vi "GTcode_v6(reorganized).vi"() -> ()   [LabVIEW 2016]
uses:
  DCScode_simulISS_MAP/flex05-4chPascal.dll
  <vilib>/Utility/config.llb/NI_LVConfig.lvlib
  <vilib>/Utility/config.llb/Write Key (U32).vi
  <vilib>/Utility/config.llb/Read Key (U32).vi
  DCScode_simulISS_MAP/flex05oem8chauto100nsPASCAL_win7.dll
  <vilib>/Analysis/NI_AALBase.lvlib
  <vilib>/Utility/config.llb/Write Key (I32).vi
  <vilib>/Utility/config.llb/Write Key (Double).vi
  <vilib>/Utility/config.llb/Write Key (String).vi
  <vilib>/Utility/config.llb/Read Key (I32).vi
panel:
  in  "Tab\nControl":T1(tab)=enum."Real Time Fitting Parameters" caption="Tab Control"
  out "filtered signal (single sample)":waveform(dbl)(graph)
  out "mean":dbl format="%0.1e"
  out "COV":dbl format="%0.1f"
  in  "Fixed Time":bool
  in  "Detector Used":T2(ring)=enum."Det 2"
  in  "Real Time Fitting?":bool=TRUE
  out "g2":cluster{"Delay Time":sgl[], sgl[]}[](graph) caption="Normalized Correlation Function"
  out "Tau":cluster{"tmp":dbl, dbl}(graph) caption="Relative Changes of Flow"
  in  "QUIT":bool
  in  "Clear plots":bool
  in  "Baseline":bool
  in  "MARK\nMark":bool
  in  "Stop":bool
  in  "Sequence Scan":bool
  out "Mark #":u32
  out "Trial #":u32
  out "Frame #":u32
  out "Det 8":sgl format="%.3f"
  out "Det 7":sgl format="%.3f"
  out "Det 6":sgl format="%.3f"
  out "Det 5":sgl format="%.3f"
  out "Det 4":sgl format="%.3f"
  out "Det 3":sgl format="%.3f"
  out "Det 2":sgl format="%.3f"
  out "Det 1":sgl format="%.3f"
  out "Computer Time":string="2010-1-12 23:16:10"
  in  "D1":bool
  in  "D2":bool
  in  "D3":bool
  in  "D4":bool
  in  "D5":bool
  in  "D6":bool
  in  "D7":bool
  in  "D8":bool
  out "Tau 2":T3(graph)={1.6593152555505744e-08, 3.9427894777554196e-08, 4.065716407938411e-08, 1.5135790977358522e-08, 2.4870420100428357e-08, 7.094765128107397e-08, 0.0, 4.1348620928852906e-07, 1.5886917674344795e-08, 4.0280526032721455e-08, -1.0, -1.0} caption="Blood Flow Index (cm2/s)"
  in  "Fixed # of Frames":u32=5
  out "Status":string="Quit"
  in  "Optical Switch OPEN":bool
  in  "Delay between frames(ms)":u32=500
  out "Time Left (ms)":sgl format="%.3f"
  in  "Integration Time (ms)":sgl=1000.0 min=1 max=13000 step=1
  in  "File Name:":string="test0"
  in  "Data Save Directory:":path=path "C:/data"
  in  "ISS Lasers ON":bool
  in  "Test":bool
  out "Data Levels":dbl(slide) scale=0.0..0.07
  in  "Lines":tag="Dev1/port1/line0:1, Dev1/port1/line3:7"
  in  "Delaytime(ms)":u32=200
  in  "Initialize Correlator":bool
  in  "Detector Select":enum32{"4 Detectors", "8 Detectors"}(radio)=enum."8 Detectors"
  in  "Update Time (ms)\nDO NOT CHANGE!":u32=105 min=1 max=999 step=1
  in  "Laser Input Name":refnum<visa-resource-name>="COM7"
  out "Flow in each detector":dbl[](array[numeric])=[-1.0, -1.0, -1.0, -1.0, -1.0, -1.0, -1.0, -1.0, -1.0, -1.0, -1.0, -1.0]
  in  "Visible\nAverages":bool[](array[boolean])=[FALSE, FALSE, FALSE, FALSE]
  in  "Avg":bool[][](array[boolean])=[[FALSE, FALSE, FALSE, FALSE, FALSE, FALSE, FALSE, FALSE], [FALSE, FALSE, FALSE, FALSE, FALSE, FALSE, FALSE, FALSE], [FALSE, FALSE, FALSE, FALSE, FALSE, FALSE, FALSE, FALSE], [FALSE, FALSE, FALSE, FALSE, FALSE, FALSE, FALSE, FALSE]]
  in  "rho":dbl[](array[numeric])=[2.5, 2.5, 2.5, 2.5, 2.5, 2.5, 2.5, 2.5, -1.0, -1.0, -1.0, -1.0]
  in  "Other Settings":u32[](array[numeric])=[1, 120, 0, 1] caption="Flow in each detector"
  in  "Initial Guess":dbl[](array[numeric])=[1e-08, 0.5, 0.05, 10.0] caption="Flow in each detector"
  out "4CH?":bool
  out "Detector#":u32=1
  out "Source#":u32=1
  # "kHz"
  # "kHz"
  # "Don't Change these Parameters unless you know clearly what you are doing"
  # "ISS Triggers Setup"
  # "Channel Parameters"
  # "Step1"
  # "Line"
  # "0"
  # "1"
  # "3"
  # "4"
  # "5"
  # "6"
  # "7"
  # "*The number of lines in the list must\nmatch the number of elements in\nthe array."
  # "Step2"
  # "Line"
  # "0"
  # "1"
  # "3"
  # "4"
  # "5"
  # "6"
  # "7"
  # "Step3"
  # "Line"
  # "0"
  # "1"
  # "3"
  # "4"
  # "5"
  # "6"
  # "7"
  # "Line    Signal\n\n0           ISS Trigger (0: OFF, 1: ON)\n1           Flow Laser 1 ON/OFF (0:OFF, 1:ON)\n2           ISS Data Acquisition (0: DONE, 1: NO)\n3           ISS Laser ON/OFF (0: ON, 1: OFF)\n4           Trigger for Marks  (0: OFF, 1: ON)\n5           Flow Laser 2 ON/OFF (0:OFF, 1:ON)\n6           Reserved\n7           Reserved"
  # "Wait ISS Data Acuisition DONE Signal"
  # "Step4"
  # "Step5"
  # "Line"
  # "0"
  # "1"
  # "3"
  # "4"
  # "5"
  # "6"
  # "7"
  # "Flow Lasers Setup"
  # "FROM FRONT PANEL"
  # "Line"
  # "0"
  # "1"
  # "3"
  # "4"
  # "5"
  # "6"
  # "7"
  # "Line"
  # "0"
  # "1"
  # "3"
  # "4"
  # "5"
  # "6"
  # "7"
  # "Det 1"
  # "Det 2"
  # "Det 3"
  # "Det 4"
  # "Det 5"
  # "Det 6"
  # "Det 7"
  # "Det 8"
  # "Avg 1"
  # "Avg 2"
  # "Avg 3"
  # "Avg 4"
  # "Db"
  # "Beta"
  # "Mua"
  # "MuS'"
  # "1"
  # "2"
  # "3"
  # "4"
  # "5"
  # "6"
  # "7"
  # "8"
  # "Avg 1"
  # "Starting Pt"
  # "End Pt"
  # "Approximate"
  # "Variables"
  # "Avg 2"
  # "Avg 3"
  # "Avg 4"
  # "Source Detector  Separations"
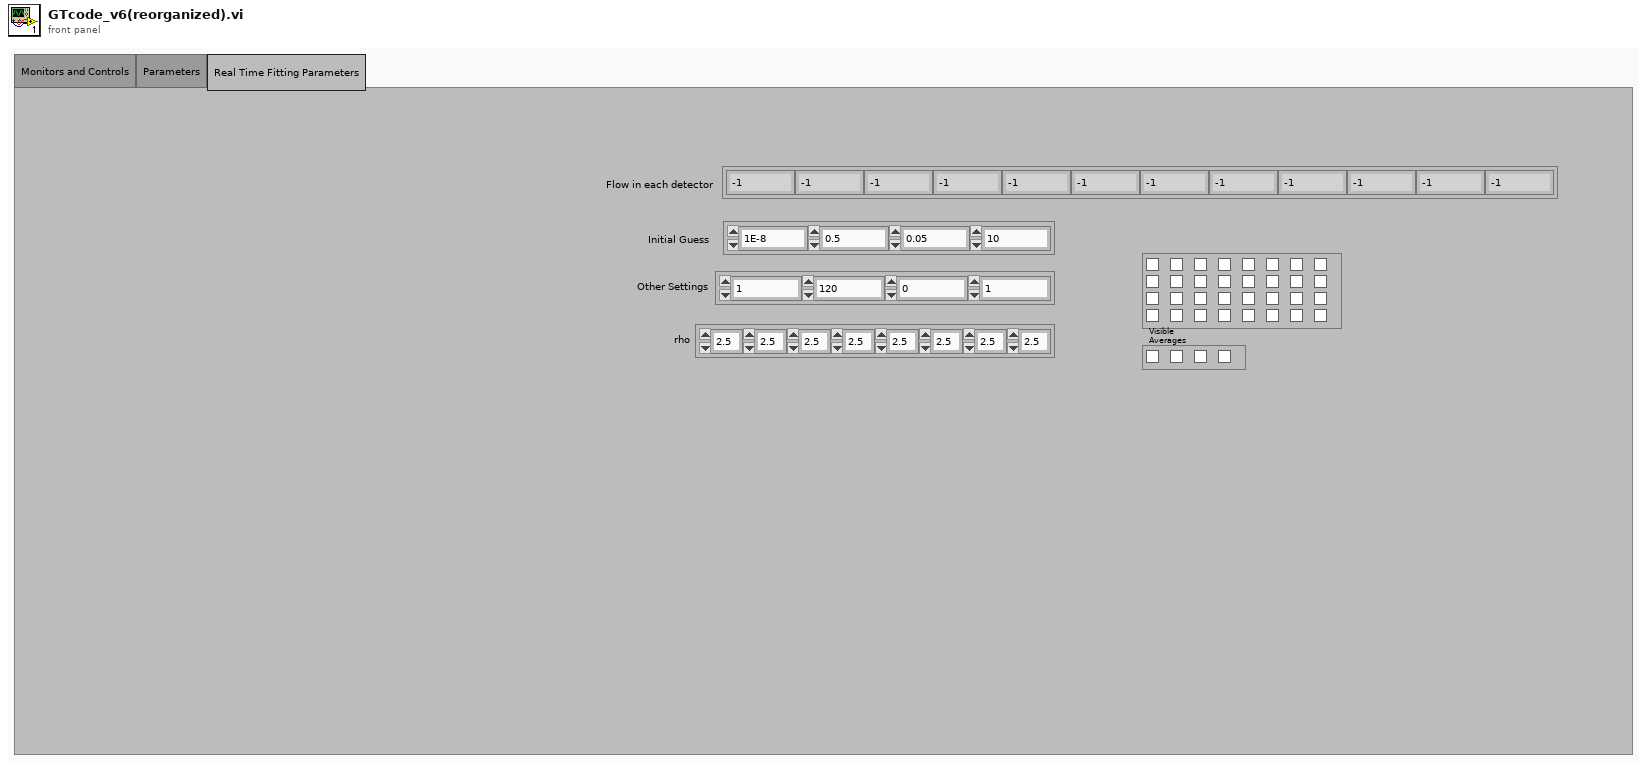
[diagram p1: front panel]
types:
  T1 = enum32{"Monitors and Controls", "Parameters", "Real Time Fitting Parameters"}
  T2 = enum16{"Det 1", "Det 2", "Det 3", "Det 4", "Det 5", "Det 6", "Det 7", "Det 8"}
  T3 = cluster{dbl, dbl, dbl, dbl, dbl, dbl, dbl, dbl, dbl, dbl, dbl, dbl}
  T4 = enum8{"Enabled", "Disabled", "Disabled and Grayed Out"}
  T5 = cluster{dbl, dbl, dbl, dbl, dbl, dbl, dbl, dbl, dbl, dbl, dbl, dbl}[]
  T6 = typedef "NI_LVConfig.lvlib/Config Data RefNum.ctl" = refnum<k1>
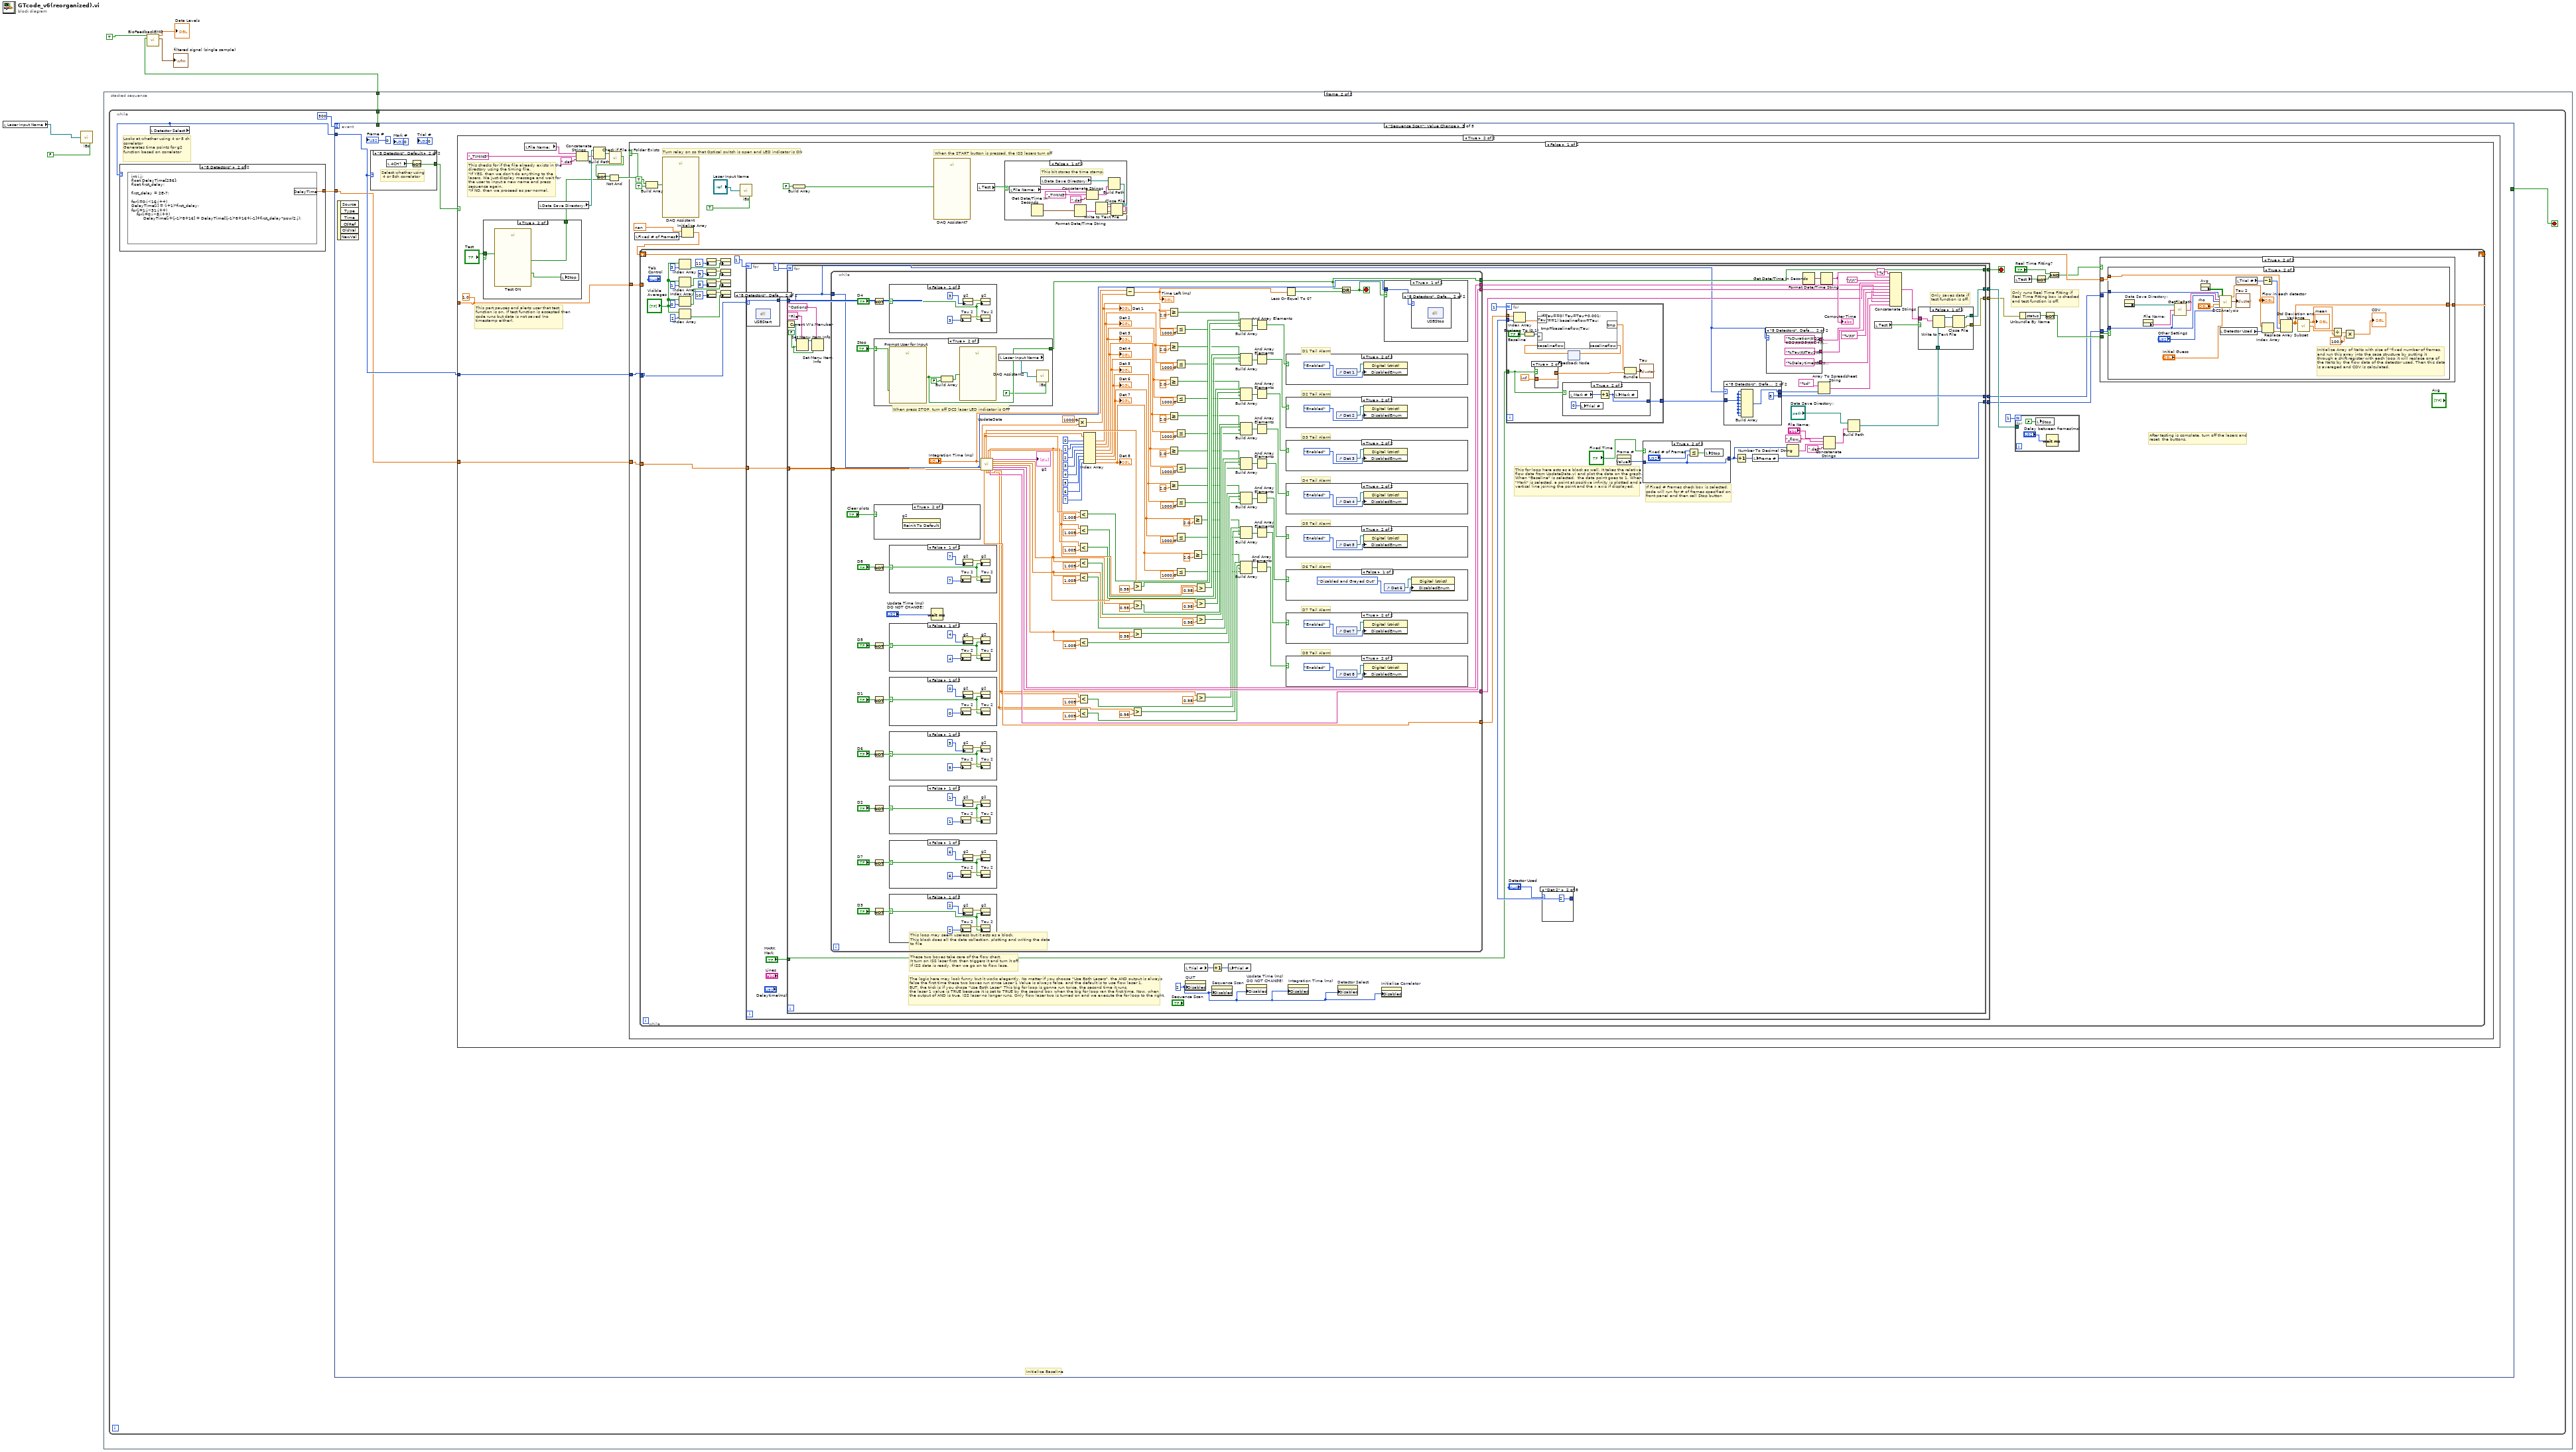
[diagram p0: block diagram]
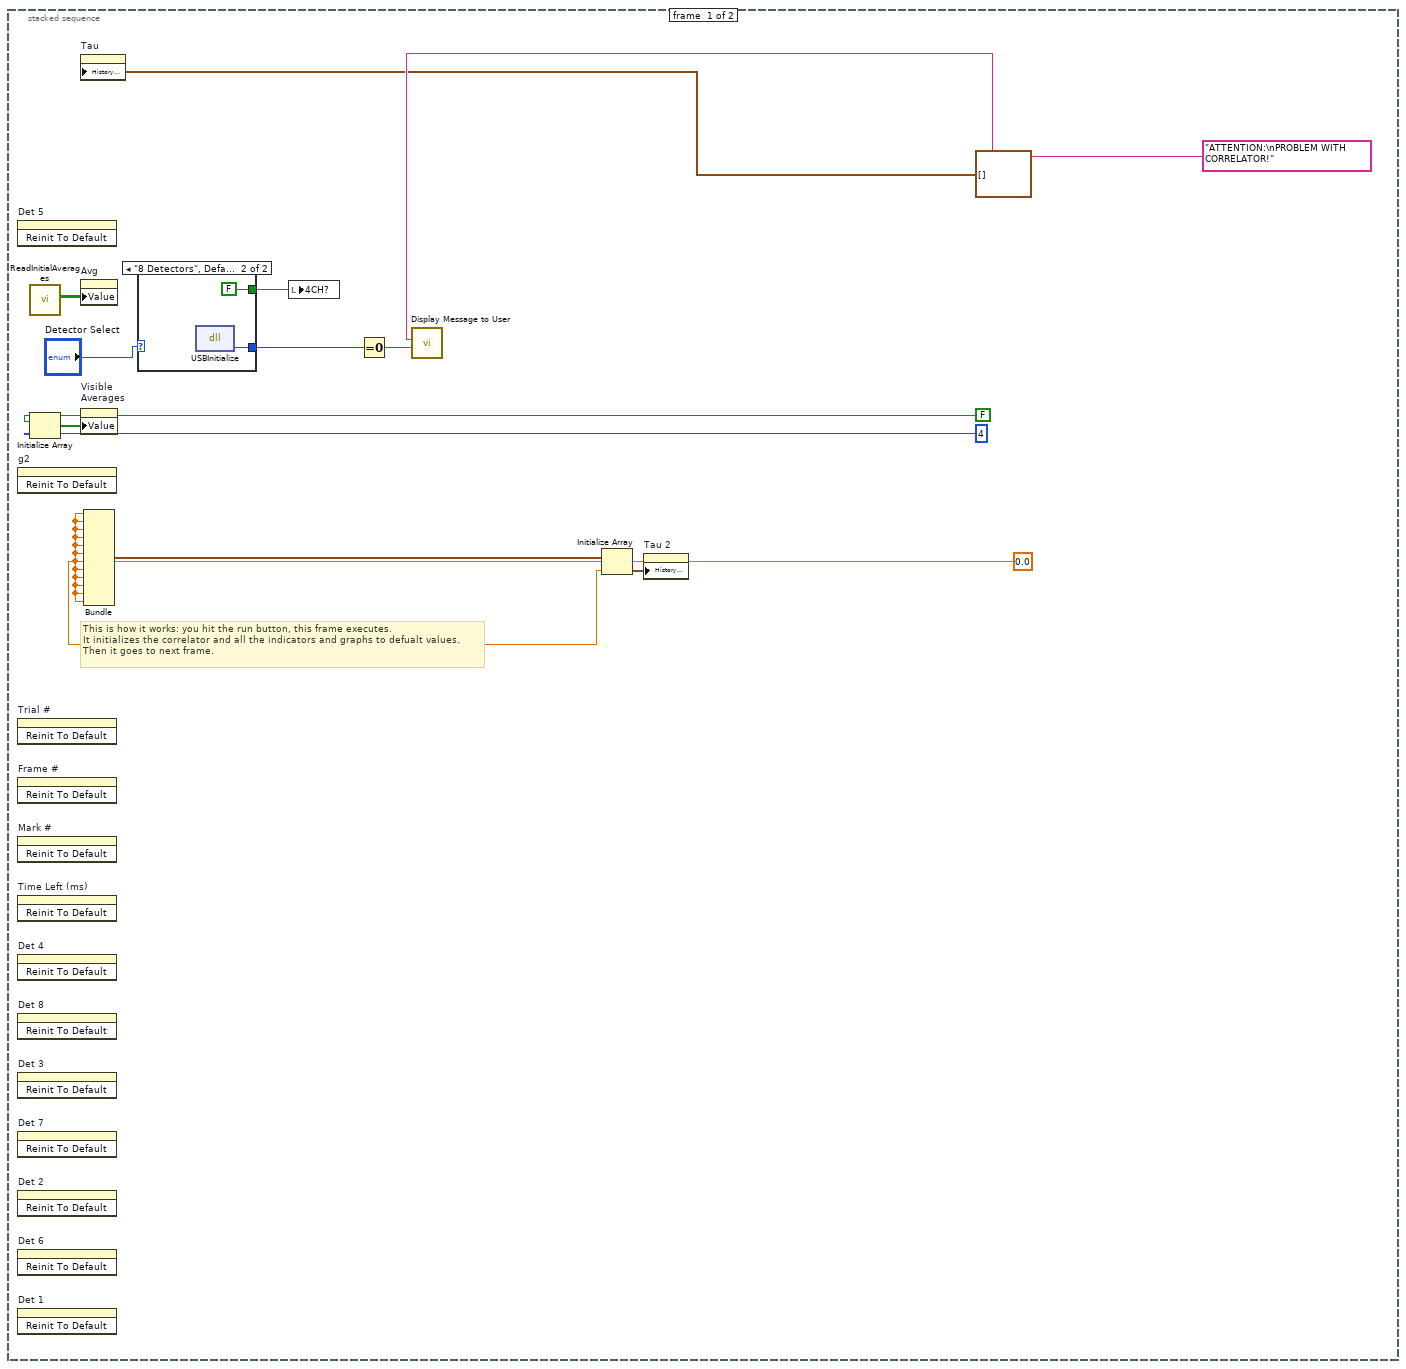
[diagram p2: hidden frame]
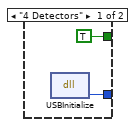
[diagram p3: hidden frame]
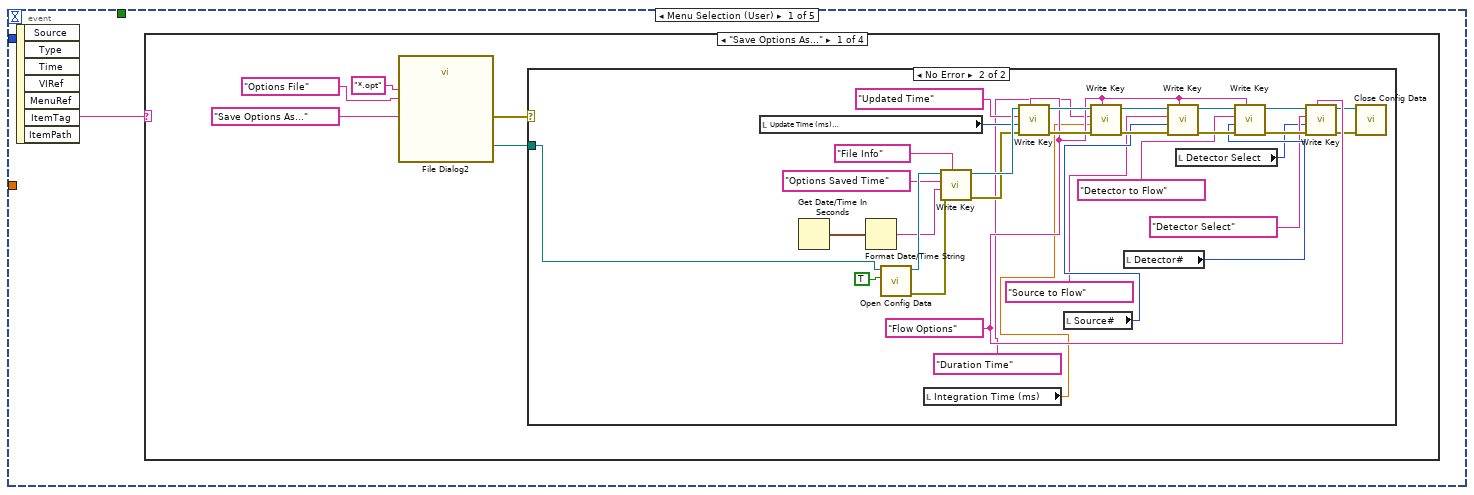
[diagram p5: hidden frame]
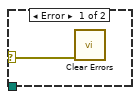
[diagram p6: hidden frame]
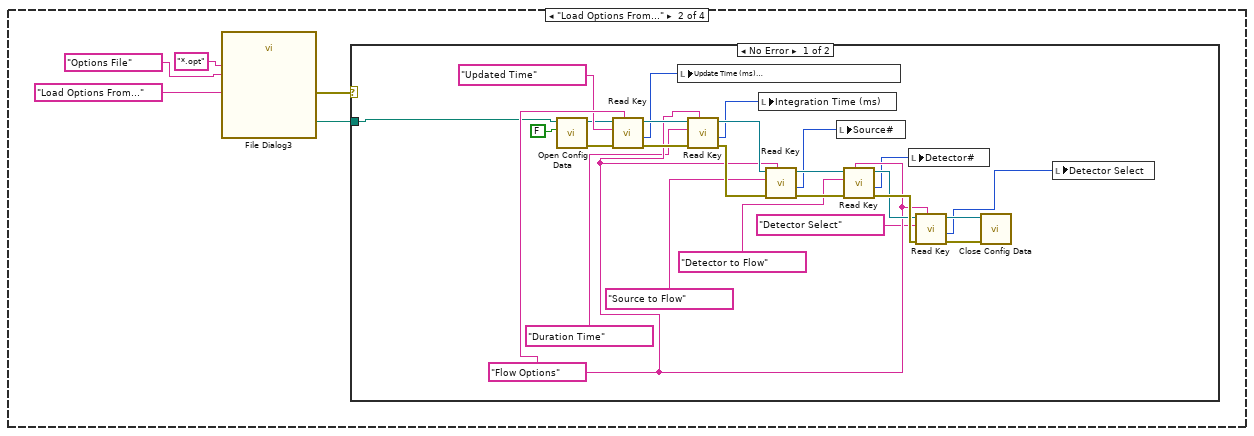
[diagram p7: hidden frame]
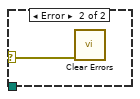
[diagram p8: hidden frame]
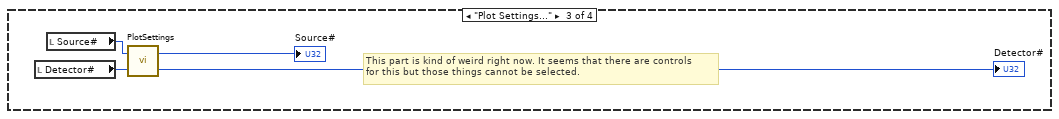
[diagram p9: hidden frame]
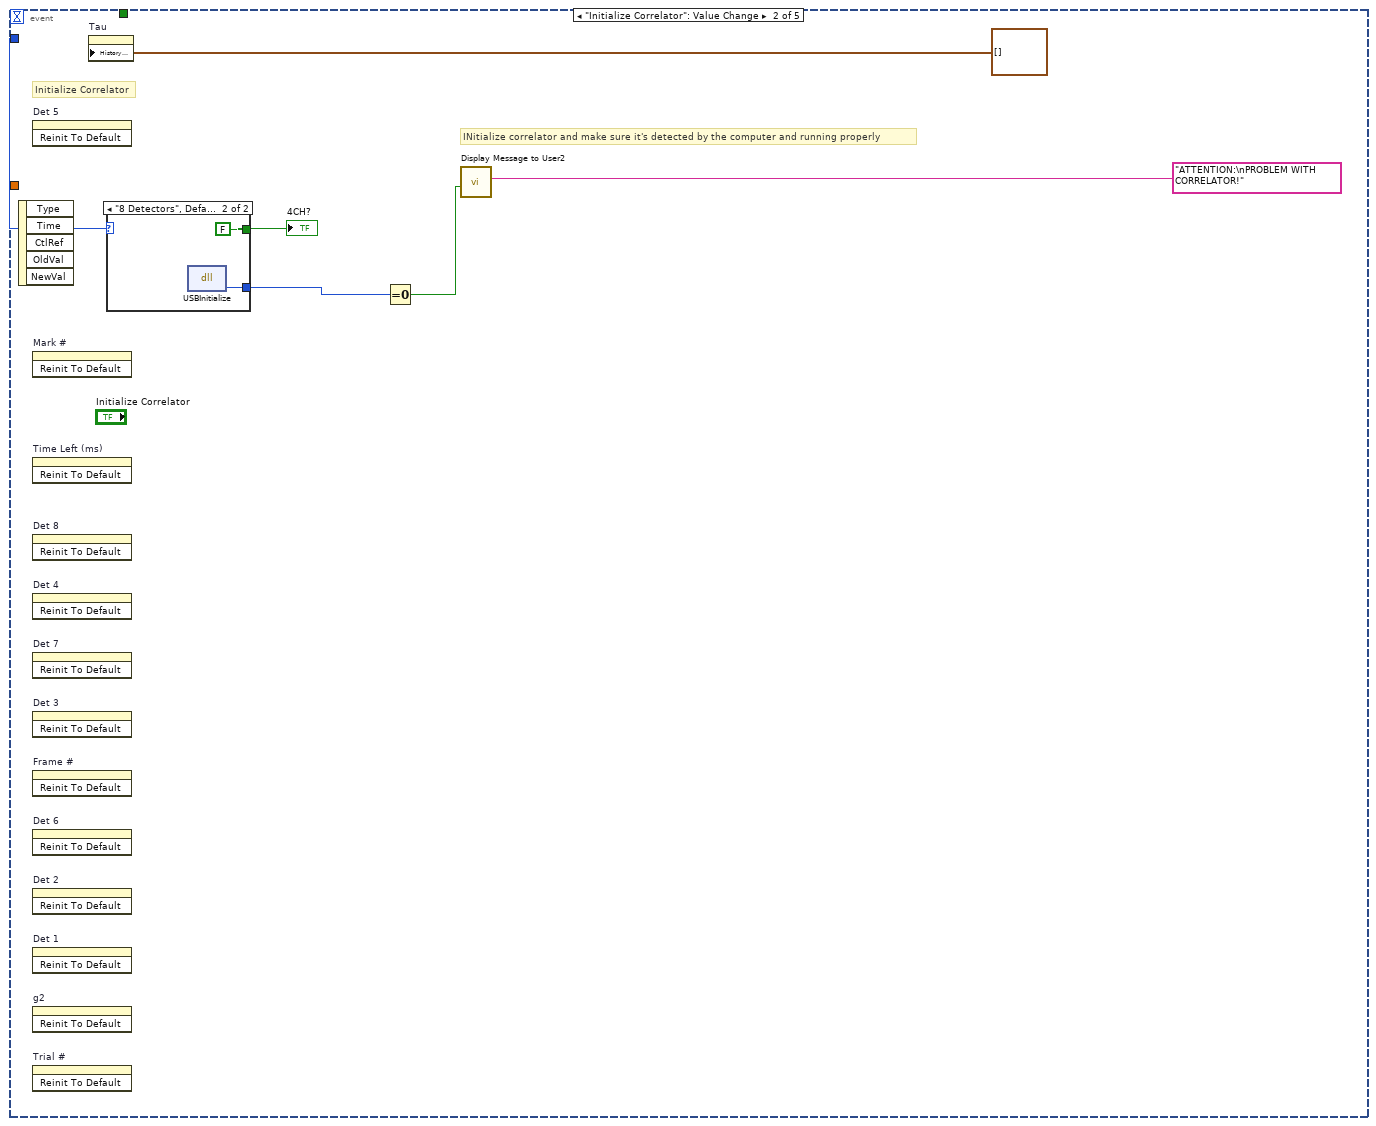
[diagram p11: hidden frame]
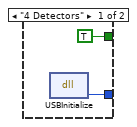
[diagram p12: hidden frame]
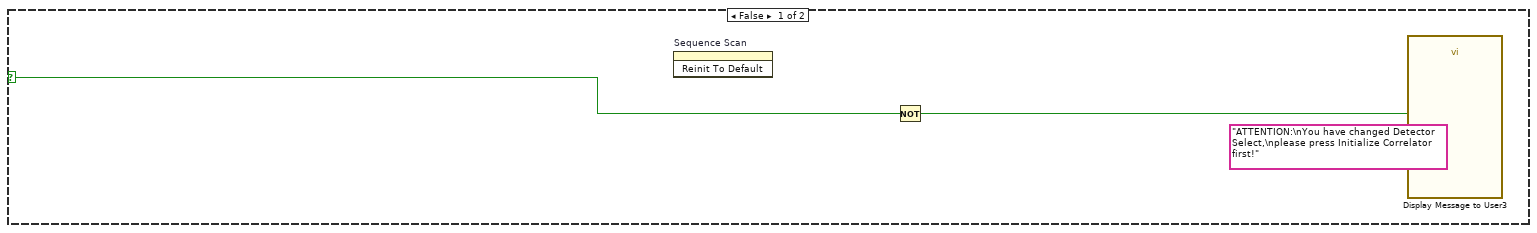
[diagram p13: hidden frame]
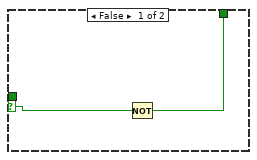
[diagram p14: hidden frame]
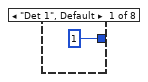
[diagram p20: hidden frame]
diagram:
  n1 = local read "Laser Input Name"() -> (w5:refnum<visa-resource-name>)
  n2 = call "iBs.vi"("Laser On/Off"=FALSE, "VISA resource name"=w5) -> ()
  n3 = stacked-sequence {
    tunnel: [_ w24] -> w2
    frame #0 {
      w9 = 0.0
      # "This is how it works: you hit the run button, this frame executes.\nIt initializes the correlator and all the indicators and graphs to defualt values.\nThen it goes to next frame."
      n4 = invoke on="Det 5" class="DigNum (strict)" method="Reinit To Default"() -> ()  [unwired: 3 in, 3 out]
      n5 = invoke on="g2" class="XYGraph (strict)" method="Reinit To Default"() -> ()  [unwired: 3 in, 3 out]
      n6 = invoke on="Trial #" class="DigNum (strict)" method="Reinit To Default"() -> ()  [unwired: 3 in, 3 out]
      n7 = invoke on="Frame #" class="DigNum (strict)" method="Reinit To Default"() -> ()  [unwired: 3 in, 3 out]
      n8 = invoke on="Mark #" class="DigNum (strict)" method="Reinit To Default"() -> ()  [unwired: 3 in, 3 out]
      n9 = invoke on="Time Left (ms)" class="DigNum (strict)" method="Reinit To Default"() -> ()  [unwired: 3 in, 3 out]
      n10 = invoke on="Det 4" class="DigNum (strict)" method="Reinit To Default"() -> ()  [unwired: 3 in, 3 out]
      n11 = invoke on="Det 8" class="DigNum (strict)" method="Reinit To Default"() -> ()  [unwired: 3 in, 3 out]
      n12 = invoke on="Det 3" class="DigNum (strict)" method="Reinit To Default"() -> ()  [unwired: 3 in, 3 out]
      n13 = invoke on="Det 7" class="DigNum (strict)" method="Reinit To Default"() -> ()  [unwired: 3 in, 3 out]
      n14 = invoke on="Det 2" class="DigNum (strict)" method="Reinit To Default"() -> ()  [unwired: 3 in, 3 out]
      n15 = invoke on="Det 6" class="DigNum (strict)" method="Reinit To Default"() -> ()  [unwired: 3 in, 3 out]
      n16 = invoke on="Det 1" class="DigNum (strict)" method="Reinit To Default"() -> ()  [unwired: 3 in, 3 out]
      n17 = call "ReadInitialAverages.vi"() -> ("avgOut"=w8:bool[][])  [unwired: 11 in]
      n18 = Initialize Array(FALSE, 4) -> (w7:bool[])
      n19 = property on="Tau" class="WFChart (strict)"("History Data"=cluster{"tmp":dbl, dbl}[] []) -> ()  [unwired: 2 in, 2 out]
      n20 = property on="Avg" class="Arr (strict)"("Value"=w8) -> ()  [unwired: 2 in, 2 out]
      n21 = property on="Visible\nAverages" class="Arr (strict)"("Value"=w7) -> ()  [unwired: 2 in, 2 out]
      n22 = Bundle(w9, w9, w9, w9, w9, w9, w9, w9, w9, w9, w9, w9) -> (w11:T3)  [unwired: 1 in]
      n23 = case shown="\"8 Detectors\", Default" "Detector Select" {
        tunnel: [w21 w23] -> w19
        tunnel: [TRUE FALSE] -> w17
        frame "4 Detectors" {
          n24 = dll-call lib="C:/Users/BUCKLEY-ADMIN/Desktop/DCScode_simulISS_MAP/flex05-4chPascal.dll" fn="USBInitialize" label="InitCH4"() -> ("return type"=w21:u8)  [unwired: 3 in, 2 out]
        }
        frame "8 Detectors", Default {
          n25 = dll-call lib="C:/Users/BUCKLEY-ADMIN/Desktop/DCScode_simulISS_MAP/flex05oem8chauto100nsPASCAL_win7.dll" fn="USBInitialize" label="InitCH8"() -> ("return type"=w23:u8)  [unwired: 3 in, 2 out]
        }
      }
      n26 = local write "4CH?"(w17) -> ()
      n27 = Equal To 0?(x=w19) -> (x = 0?=w18:bool)
      n28 = call "Display Message to User"("Enable"=w18, "Message"="ATTENTION:\nPROBLEM WITH CORRELATOR!") -> ()  [unwired: 8 in, 2 out]
      n29 = Initialize Array(w11, w9) -> (w10:T5)
      n30 = property on="Tau 2" class="WFChart (strict)"("History Data"=w10) -> ()  [unwired: 2 in, 2 out]
    }
    frame #1 {
      n31 = while {
        tunnel: [w25] -> w24
        stop <- w26 stop-if-true
        # "Looks at whether using 4 or 8 ch correlator\nGenerates time points for g2 function based on correlator"
        n32 = local read "Detector Select"() -> (w27:enum32{"4 Detectors", "8 Detectors"})
        n33 = case shown="\"8 Detectors\"" w27 {
          tunnel: [_ w30] -> w28
          frame "4 Detectors", Default {
          }
          frame "8 Detectors" {
            n34 = formula code="int i,j;\nfloat DelayTime[256];\nfloat first_delay;\n\nfirst_delay = 2E-7;\n\nfor(i=0;i<16;i++)\nDelayTime[i] = (i+1)*first_delay;\nfor(j=1;j<31;j++)\n    for(i=0;i<8;i++)\n         DelayTime[i+(j-1)*8+16] = DelayTime[(j-1)*8+16+i-1]+first_delay*pow(2,j);"() -> ("DelayTime"=w30:dbl[])
          }
        }
        n35 = event shown="[2] \"Sequence Scan\": Value Change" {
          selector: _ -> [_ _ _ _ _]
          dyn-events: _ -> [_ _ _ _ _]
          timeout: 500 -> [_ _ _ _ _]
          tunnel: w28 -> [_ _ w114 _ _]
          tunnel: [_ _ _ "QUIT" _] -> w26
          tunnel: w27 -> [_ w107 w115 w604 _]
          tunnel: [_ _ _ "QUIT" _] -> w25
          event Menu Selection (User) {
            n36 = event-data() -> ("ItemTag"=w31:string)  [unwired: 1 in, 6 out]
            n37 = case shown="\"Save Options As...\"" w31 {
              frame "Save Options As..." {
                n38 = call "File Dialog2"("prompt"="Save Options As...", "pattern (all files)"="*.opt", "pattern label"="Options File") -> ("selected path"=w33:path, "error out"=w32:errorcluster)  [unwired: 9 in, 2 out]
                n39 = case shown="No Error" w32 {
                  selector: w32 -> [w37 _]
                  tunnel: w33 -> [_ w68]
                  frame Error {
                    n40 = call <vilib>:"Clear Errors.vi"("error in (no error)"=w37) -> ()  [unwired: 5 in, 2 out]
                  }
                  frame No Error {
                    w55 = "Flow Options"
                    n41 = local read "Update Time (ms)\nDO NOT CHANGE!"() -> (w48:u32)
                    n42 = Get Date/Time In Seconds() -> (seconds since 1Jan1904=w54:timestamp)
                    n43 = Format Date/Time String(seconds (now)=w54) -> (date/time string=w50:string)  [unwired: 2 in]
                    n44 = call <vilib>:"Open Config Data.vi"("create file if necessary (T)"=TRUE, "configuration file path"=w68) -> ("error out"=w66:errorcluster, "refnum"=w65:T6)  [unwired: 7 in, 1 out]
                    n45 = local read "Integration Time (ms)"() -> (w46:sgl)
                    n46 = call-poly <vilib>:"Write Key.vi"("section"="File Info", "error in (no error)"=w66, "value"=w50, "key"="Options Saved Time", "refnum"=w65) -> ("error out"=w52:errorcluster, "refnum out"=w53:T6)  [unwired: 4 in, 1 out]
                    n47 = call-poly <vilib>:"Write Key.vi"("section"=w55, "error in (no error)"=w52, "value"=w48, "key"="Updated Time", "refnum"=w53) -> ("error out"=w64:errorcluster, "refnum out"=w63:T6)  [unwired: 4 in, 1 out]
                    n48 = local read "Source#"() -> (w45:u32)
                    n49 = call-poly <vilib>:"Write Key.vi"("section"=w55, "error in (no error)"=w64, "value"=w46, "key"="Duration Time", "refnum"=w63) -> ("error out"=w59:errorcluster, "refnum out"=w60:T6)  [unwired: 4 in, 1 out]
                    n50 = local read "Detector#"() -> (w42:u32)
                    n51 = call-poly <vilib>:"Write Key.vi"("section"=w55, "error in (no error)"=w59, "value"=w45, "key"="Source to Flow", "refnum"=w60) -> ("error out"=w61:errorcluster, "refnum out"=w62:T6)  [unwired: 4 in, 1 out]
                    n52 = local read "Detector Select"() -> (w40:enum32{"4 Detectors", "8 Detectors"})
                    n53 = call-poly <vilib>:"Write Key.vi"("section"=w55, "error in (no error)"=w61, "value"=w42, "key"="Detector to Flow", "refnum"=w62) -> ("error out"=w58:errorcluster, "refnum out"=w57:T6)  [unwired: 4 in, 1 out]
                    n54 = call-poly <vilib>:"Write Key.vi"("section"=w55, "error in (no error)"=w58, "value"=w40, "key"="Detector Select", "refnum"=w57) -> ("error out"=w38:errorcluster, "refnum out"=w39:T6)  [unwired: 4 in, 1 out]
                    n55 = call <vilib>:"Close Config Data.vi"("error in (no error)"=w38, "refnum"=w39) -> ()  [unwired: 8 in, 2 out]
                  }
                }
              }
              frame "Load Options From..." {
                n56 = call "File Dialog3"("prompt"="Load Options From...", "pattern (all files)"="*.opt", "pattern label"="Options File") -> ("selected path"=w70:path, "error out"=w69:errorcluster)  [unwired: 9 in, 2 out]
                n57 = case shown="No Error" w69 {
                  selector: w69 -> [_ w99]
                  tunnel: w70 -> [w74 _]
                  frame No Error {
                    w89 = "Flow Options"
                    n58 = call <vilib>:"Open Config Data.vi"("create file if necessary (T)"=FALSE, "configuration file path"=w74) -> ("error out"=w81:errorcluster, "refnum"=w80:T6)  [unwired: 7 in, 1 out]
                    n59 = call-poly <vilib>:"Read Key.vi"("section"=w89, "error in (no error)"=w81, "key"="Updated Time", "refnum"=w80) -> ("error out"=w97:errorcluster, "value"=w79:u32, "refnum out"=w96:T6)  [unwired: 4 in, 1 out]
                    n60 = local write "Update Time (ms)\nDO NOT CHANGE!"(w79) -> ()
                    n61 = call-poly <vilib>:"Read Key.vi"("section"=w89, "error in (no error)"=w97, "key"="Duration Time", "refnum"=w96) -> ("error out"=w92:errorcluster, "value"=w78:i32, "refnum out"=w93:T6)  [unwired: 4 in, 1 out]
                    n62 = local write "Integration Time (ms)"(w78) -> ()
                    n63 = call-poly <vilib>:"Read Key.vi"("section"=w89, "error in (no error)"=w92, "key"="Source to Flow", "refnum"=w93) -> ("error out"=w94:errorcluster, "value"=w75:u32, "refnum out"=w95:T6)  [unwired: 4 in, 1 out]
                    n64 = local write "Source#"(w75) -> ()
                    n65 = call-poly <vilib>:"Read Key.vi"("section"=w89, "error in (no error)"=w94, "key"="Detector to Flow", "refnum"=w95) -> ("error out"=w91:errorcluster, "value"=w76:u32, "refnum out"=w90:T6)  [unwired: 4 in, 1 out]
                    n66 = local write "Detector#"(w76) -> ()
                    n67 = call-poly <vilib>:"Read Key.vi"("section"=w89, "error in (no error)"=w91, "key"="Detector Select", "refnum"=w90) -> ("error out"=w82:errorcluster, "value"=w77:u32, "refnum out"=w83:T6)  [unwired: 4 in, 1 out]
                    n68 = call <vilib>:"Close Config Data.vi"("error in (no error)"=w82, "refnum"=w83) -> ()  [unwired: 8 in, 2 out]
                    n69 = local write "Detector Select"(w77) -> ()
                  }
                  frame Error {
                    n70 = call <vilib>:"Clear Errors.vi"("error in (no error)"=w99) -> ()  [unwired: 5 in, 2 out]
                  }
                }
              }
              frame "Plot Settings..." {
                # "This part is kind of weird right now. It seems that there are controls\nfor this but those things cannot be selected."
                n71 = local read "Detector#"() -> (w101:u32)
                n72 = local read "Source#"() -> (w102:u32)
                n73 = call "PlotSettings.vi"("Detectorin"=w101, "Sourcein"=w102) -> ("Detector#"=→"Detector#":u32, "Source#"=→"Source#":u32)
              }
              frame Default {
              }
            }
          }
          event "Initialize Correlator": Value Change {
            # "INitialize correlator and make sure it's detected by the computer and running properly"
            # "Initialize Correlator"
            n74 = event-data() -> ()  [unwired: 1 in, 5 out]
            n75 = invoke on="Det 5" class="DigNum (strict)" method="Reinit To Default"() -> ()  [unwired: 3 in, 3 out]
            n76 = invoke on="Mark #" class="DigNum (strict)" method="Reinit To Default"() -> ()  [unwired: 3 in, 3 out]
            n77 = invoke on="Time Left (ms)" class="DigNum (strict)" method="Reinit To Default"() -> ()  [unwired: 3 in, 3 out]
            n78 = invoke on="Det 8" class="DigNum (strict)" method="Reinit To Default"() -> ()  [unwired: 3 in, 3 out]
            n79 = invoke on="Det 4" class="DigNum (strict)" method="Reinit To Default"() -> ()  [unwired: 3 in, 3 out]
            n80 = invoke on="Det 7" class="DigNum (strict)" method="Reinit To Default"() -> ()  [unwired: 3 in, 3 out]
            n81 = invoke on="Det 3" class="DigNum (strict)" method="Reinit To Default"() -> ()  [unwired: 3 in, 3 out]
            n82 = invoke on="Frame #" class="DigNum (strict)" method="Reinit To Default"() -> ()  [unwired: 3 in, 3 out]
            n83 = invoke on="Det 6" class="DigNum (strict)" method="Reinit To Default"() -> ()  [unwired: 3 in, 3 out]
            n84 = invoke on="Det 2" class="DigNum (strict)" method="Reinit To Default"() -> ()  [unwired: 3 in, 3 out]
            n85 = invoke on="Det 1" class="DigNum (strict)" method="Reinit To Default"() -> ()  [unwired: 3 in, 3 out]
            n86 = invoke on="g2" class="XYGraph (strict)" method="Reinit To Default"() -> ()  [unwired: 3 in, 3 out]
            n87 = invoke on="Trial #" class="DigNum (strict)" method="Reinit To Default"() -> ()  [unwired: 3 in, 3 out]
            n88 = property on="Tau" class="WFChart (strict)"("History Data"=cluster{"tmp":dbl, dbl}[] []) -> ()  [unwired: 2 in, 2 out]
            n89 = case shown="\"8 Detectors\", Default" w107 {
              tunnel: [w111 w113] -> w109
              tunnel: [TRUE FALSE] -> w106
              frame "4 Detectors" {
                n90 = dll-call lib="C:/Users/BUCKLEY-ADMIN/Desktop/DCScode_simulISS_MAP/flex05-4chPascal.dll" fn="USBInitialize" label="InitCH4"() -> ("return type"=w111:u8)  [unwired: 3 in, 2 out]
              }
              frame "8 Detectors", Default {
                n91 = dll-call lib="C:/Users/BUCKLEY-ADMIN/Desktop/DCScode_simulISS_MAP/flex05oem8chauto100nsPASCAL_win7.dll" fn="USBInitialize" label="InitCH8"() -> ("return type"=w113:u8)  [unwired: 3 in, 2 out]
              }
            }
            "4CH?" <- w106
            n92 = Equal To 0?(x=w109) -> (x = 0?=w108:bool)
            n93 = call "Display Message to User2"("Enable"=w108, "Message"="ATTENTION:\nPROBLEM WITH CORRELATOR!") -> ()  [unwired: 8 in, 2 out]
          }
          event "Sequence Scan": Value Change {
            # "Initialize Baseline"
            n94 = event-data() -> ()  [unwired: 1 in, 6 out]
            n95 = case shown="\"8 Detectors\", Default" w115 {
              tunnel: [w598 w599] -> w116
              frame "4 Detectors" {
                n96 = local read "4CH?"() -> (w598:bool)
              }
              frame "8 Detectors", Default {
                # "Select whether using\n 4 or 8ch correlator"
                n97 = local read "4CH?"() -> (w600:bool)
                n98 = Not(x=w600) -> (.not. x?=w599:bool)
              }
            }
            n99 = case shown="True" w116 {
              selector: w116 -> [w121 _]
              tunnel: w114 -> [_ w135]
              tunnel: w115 -> [_ w136]
              tunnel: [_ w123] -> _
              frame False {
                n100 = invoke on="Sequence Scan" class="Bool" method="Reinit To Default"() -> ()  [unwired: 3 in, 3 out]
                n101 = Not(x=w121) -> (.not. x?=w120:bool)
                n102 = call "Display Message to User3"("Enable"=w120, "Message"="ATTENTION:\nYou have changed Detector Select,\nplease press Initialize Correlator first!") -> ()  [unwired: 8 in, 2 out]
              }
              frame True {
                w123 = sgl 1.0
                # "This part pauses and alerts user that test function is on. If test function is accepted then code runs but data is not saved (no timestamp either)."
                # "This checks for if the file already exists in the directory using the timing file. \n*If YES, then we don't do anything to the lasers. We just display message and wait for the user to input a new name and press sequence again.\n*If NO, then we proceed as per normal."
                n103 = case shown="True" "Test" {
                  selector: "Test" -> [w138 _]
                  tunnel: "Test" -> [_ w140]
                  tunnel: [w137 w139] -> w124
                  frame False {
                    n104 = Not(x=w138) -> (.not. x?=w137:bool)
                  }
                  frame True {
                    n105 = call "Test ON"("Enable"=w140) -> ("No - STOP"=w141:bool, "OK"=w139:bool)  [unwired: 15 in, 2 out]
                    n106 = local write "Stop"(w141) -> ()
                  }
                }
                n107 = local read "File Name:"() -> (w131:string)
                n108 = local read "Data Save Directory:"() -> (w130:path)
                n109 = Concatenate Strings(w131, "_TIMING", ".dat") -> (w133:string)
                n110 = Build Path(base path=w130, name or relative path=w133) -> (appended path=w129:path)
                n111 = call <vilib>:"Check if File or Folder Exists.vi"("path"=w129) -> ("file or folder exists?"=w126:bool)  [unwired: 8 in, 2 out]
                n112 = Not(x=w126) -> (.not. x?=w128:bool)
                n113 = Not And(1:w124, 2:w128) -> (0:w127:bool)
                n114 = case shown="False" w127 {
                  tunnel: w136 -> [w143 _]
                  tunnel: w135 -> [w144 _]
                  tunnel: w123 -> [w145 _]
                  frame False {
                    # "Turn relay on so that Optical switch is open and LED indicator is ON"
                    # "When the START button is pressed, the ISS lasers turn off"
                    n115 = local read "Fixed # of Frames"() -> (w150:u32)
                    n116 = Build Array(TRUE, TRUE) -> (w155:bool[])
                    n117 = call "DAQ Assistant"("data"=w155) -> ()  [unwired: 17 in, 2 out]
                    n118 = Initialize Array "Initialize Array"(nan, w150) -> (w142:dbl[])
                    n119 = while {
                      tunnel: w143 -> [w169]
                      tunnel: w144 -> [w199]
                      tunnel: w145 -> [_]
                      shift-right: [w172] -> _
                      shift-left: w142 -> [w173]
                      stop <- w174 stop-if-true
                      # "Only runs Real Time Fitting if \nReal Time Fitting box is checked \nand test function is off."
                      # "After testing is complete, turn off the lasers and\nreset  the buttons."
                      n120 = Index Array(array="Visible\nAverages", index=3) -> (element=w192:bool)
                      n121 = Index Array(array="Visible\nAverages", index=1) -> (element=w193:bool)
                      n122 = Index Array(array="Visible\nAverages", index=0) -> (element=w186:bool)
                      n123 = Index Array(array="Visible\nAverages", index=2) -> (element=w187:bool)
                      n124 = property on="Tau 2" class="WFChart (strict)"("Active Plot"=u32 11) -> (error out=w190:errorcluster)  [unwired: 2 in, 1 out]
                      n125 = property on="Tau 2" class="WFChart (strict)"("Active Plot"=u32 9) -> (error out=w195:errorcluster)  [unwired: 2 in, 1 out]
                      n126 = property on="Tau 2" class="WFChart (strict)"("Active Plot"=u32 8) -> (error out=w184:errorcluster)  [unwired: 2 in, 1 out]
                      n127 = property on="Tau 2" class="WFChart (strict)"("Active Plot"=u32 10) -> (error out=w189:errorcluster)  [unwired: 2 in, 1 out]
                      n128 = property on="Tau 2" class="WFChart (strict)"(error in=w190, "Plot.Visible?"=w192) -> ()  [unwired: 1 in, 2 out]
                      n129 = property on="Tau 2" class="WFChart (strict)"(error in=w195, "Plot.Visible?"=w193) -> ()  [unwired: 1 in, 2 out]
                      n130 = property on="Tau 2" class="WFChart (strict)"(error in=w184, "Plot.Visible?"=w186) -> ()  [unwired: 1 in, 2 out]
                      n131 = property on="Tau 2" class="WFChart (strict)"(error in=w189, "Plot.Visible?"=w187) -> ()  [unwired: 1 in, 2 out]
                      n132 = for {
                        N: 1 -> [_]
                        tunnel: w199 -> [w240]
                        tunnel: w169 -> [w239]
                        tunnel: [w236] -> w174
                        tunnel: [w235] -> w198
                        tunnel: [w233] -> w178
                        tunnel: [w231] -> w177
                        tunnel: [w232] -> w176
                        # "The logic here may look funny but it works elegantly. No matter if you choose \"Use Both Lasers\", the AND output is always\nfalse the first time these two boxes run since Laser 1 Value is always false, and the default is to use flow laser 1.\nBUT, the trick is if you chose \"Use Both Laser\" This big for loop is gonna run twice, the second time it runs, \nthe laser 1 value is TRUE because it is set to TRUE by the second box when the big for loop ran the first time. Now, when\nthe output of AND is true, ISS laser no longer runs. Only flow laser two is turned on and we execute the for loop to the right."
                        # "These two boxes take care of the flow chart.\nIt turn on ISS laser first, then triggers it and turn it off.\nIf ISS data is ready, then we go on to flow lase."
                        # "This loop may seem useless but it acts as a block. \nThis block does all the data collection, plotting and writing the data\nto file"
                        n133 = case shown="\"8 Detectors\", Default" w239 {
                          selector: w239 -> [w596 w597]
                          tunnel: [w596 w597] -> w237
                          frame "4 Detectors" {
                            n134 = dll-call lib="C:/Users/BUCKLEY-ADMIN/Desktop/DCScode_simulISS_MAP/flex05-4chPascal.dll" fn="USBStart" label="StartCH4"() -> ()  [unwired: 4 in, 2 out]
                          }
                          frame "8 Detectors", Default {
                            n135 = dll-call lib="C:/Users/BUCKLEY-ADMIN/Desktop/DCScode_simulISS_MAP/flex05oem8chauto100nsPASCAL_win7.dll" fn="USBStart" label="StartCH8"() -> ()  [unwired: 4 in, 2 out]
                          }
                        }
                        n136 = for {
                          N: 1 -> [_]
                          tunnel: w240 -> [w264]
                          tunnel: [w244] -> w236
                          tunnel: w237 -> [w241]
                          tunnel: [w246] -> w235
                          tunnel: "MARK\nMark" -> [w258]
                          tunnel: [w245] -> w233
                          tunnel: [w243] -> w231
                          tunnel: [w257] -> w232
                          w250 = FALSE
                          w242 = u8 2
                          # "Only saves data if\ntest function is off."
                          # "If Fixed # Frames check box is selected,\ncode will run for # of frames specified on \nfront panel and then call Stop button"
                          # "This for loop here acts as a block as well. It takes the relative \nflow data from UpdateData.vi and plot the data on the graph.\nWhen \"Baseline\" is selected,  the data point goes to 1. When\n\"Mark\" is selected, a point at positive infinity is plotted and a\nvertical line joining the point and the x axis if displayed."
                          n137 = Current VI's Menubar() -> (w266:refnum<k9>)
                          n138 = Set Menu Item Info(7:"File", 9:w250, 11:w266) -> (3:w265:refnum<k9>)  [unwired: 4 in, 1 out]
                          n139 = Set Menu Item Info(7:"Options", 9:w250, 11:w265) -> ()  [unwired: 4 in, 2 out]
                          n140 = while {
                            tunnel: [w452] -> w272
                            tunnel: [w422] -> w271
                            tunnel: [w423] -> w270
                            tunnel: [w426] -> w244
                            tunnel: [w453] -> w269
                            tunnel: w264 -> [w455]
                            tunnel: w241 -> [w428]
                            stop <- w457 stop-if-true
                            # "D4 Tail Alarm"
                            # "D2 Tail Alarm"
                            # "D8 Tail Alarm"
                            # "D7 Tail Alarm"
                            # "D6 Tail Alarm"
                            # "D5 Tail Alarm"
                            # "D3 Tail Alarm"
                            # "D1 Tail Alarm"
                            # "When press STOP, turn off DCS laser LED indicator is OFF"
                            n141 = Not(x="D4") -> (.not. x?=w441:bool)
                            n142 = Not(x="D8") -> (.not. x?=w437:bool)
                            n143 = Not(x="D5") -> (.not. x?=w440:bool)
                            n144 = Not(x="D1") -> (.not. x?=w444:bool)
                            n145 = Not(x="D6") -> (.not. x?=w439:bool)
                            n146 = Not(x="D2") -> (.not. x?=w429:bool)
                            n147 = Not(x="D7") -> (.not. x?=w438:bool)
                            n148 = Not(x="D3") -> (.not. x?=w442:bool)
                            n149 = case shown="True" "Stop" {
                              selector: "Stop" -> [w496 w502]
                              tunnel: [w496 w499] -> w426
                              frame False {
                              }
                              frame True {
                                n150 = call "Prompt User for Input"("Enable"=w502) -> ("Yes"=w499:bool)  [unwired: 17 in, 1 out]
                                n151 = Build Array(w499, FALSE) -> (w501:bool[])
                                n152 = call "DAQ Assistant2"("data"=w501) -> ()  [unwired: 17 in, 2 out]
                                n153 = local read "Laser Input Name"() -> (w497:refnum<visa-resource-name>)
                                n154 = call "iBs.vi"("Laser On/Off"=FALSE, "VISA resource name"=w497) -> ()
                              }
                            }
                            n155 = case shown="True" "Clear plots" {
                              frame False {
                              }
                              frame True {
                                n156 = invoke on="g2" class="XYGraph (strict)" method="Reinit To Default"() -> ()  [unwired: 3 in, 3 out]
                              }
                            }
                            n157 = case shown="False" w441 {
                              selector: w441 -> [w543 w548]
                              frame False {
                                n158 = property on="Tau 2" class="WFChart (strict)"("Active Plot"=u32 3) -> (error out=w545:errorcluster)  [unwired: 2 in, 1 out]
                                n159 = property on="g2" class="XYGraph (strict)"("Active Plot"=u32 3) -> (error out=w546:errorcluster)  [unwired: 2 in, 1 out]
                                n160 = property on="g2" class="XYGraph (strict)"(error in=w546, "Plot.Visible?"=w543) -> ()  [unwired: 1 in, 2 out]
                                n161 = property on="Tau 2" class="WFChart (strict)"(error in=w545, "Plot.Visible?"=w543) -> ()  [unwired: 1 in, 2 out]
                              }
                              frame True {
                                n162 = property on="Tau 2" class="WFChart (strict)"("Active Plot"=u32 3) -> (error out=w549:errorcluster)  [unwired: 2 in, 1 out]
                                n163 = property on="Tau 2" class="WFChart (strict)"(error in=w549, "Plot.Visible?"=w548) -> ()  [unwired: 1 in, 2 out]
                                n164 = property on="g2" class="XYGraph (strict)"("Active Plot"=u32 3) -> (error out=w551:errorcluster)  [unwired: 2 in, 1 out]
                                n165 = property on="g2" class="XYGraph (strict)"(error in=w551, "Plot.Visible?"=w548) -> ()  [unwired: 1 in, 2 out]
                              }
                            }
                            n166 = case shown="False" w437 {
                              selector: w437 -> [w503 w508]
                              frame False {
                                n167 = property on="Tau 2" class="WFChart (strict)"("Active Plot"=u32 7) -> (error out=w504:errorcluster)  [unwired: 2 in, 1 out]
                                n168 = property on="g2" class="XYGraph (strict)"("Active Plot"=u32 7) -> (error out=w506:errorcluster)  [unwired: 2 in, 1 out]
                                n169 = property on="g2" class="XYGraph (strict)"(error in=w506, "Plot.Visible?"=w503) -> ()  [unwired: 1 in, 2 out]
                                n170 = property on="Tau 2" class="WFChart (strict)"(error in=w504, "Plot.Visible?"=w503) -> ()  [unwired: 1 in, 2 out]
                              }
                              frame True {
                                n171 = property on="Tau 2" class="WFChart (strict)"("Active Plot"=u32 7) -> (error out=w510:errorcluster)  [unwired: 2 in, 1 out]
                                n172 = property on="Tau 2" class="WFChart (strict)"(error in=w510, "Plot.Visible?"=w508) -> ()  [unwired: 1 in, 2 out]
                                n173 = property on="g2" class="XYGraph (strict)"("Active Plot"=u32 7) -> (error out=w511:errorcluster)  [unwired: 2 in, 1 out]
                                n174 = property on="g2" class="XYGraph (strict)"(error in=w511, "Plot.Visible?"=w508) -> ()  [unwired: 1 in, 2 out]
                              }
                            }
                            n175 = case shown="False" w440 {
                              selector: w440 -> [w533 w538]
                              frame False {
                                n176 = property on="Tau 2" class="WFChart (strict)"("Active Plot"=u32 4) -> (error out=w535:errorcluster)  [unwired: 2 in, 1 out]
                                n177 = property on="g2" class="XYGraph (strict)"("Active Plot"=u32 4) -> (error out=w536:errorcluster)  [unwired: 2 in, 1 out]
                                n178 = property on="g2" class="XYGraph (strict)"(error in=w536, "Plot.Visible?"=w533) -> ()  [unwired: 1 in, 2 out]
                                n179 = property on="Tau 2" class="WFChart (strict)"(error in=w535, "Plot.Visible?"=w533) -> ()  [unwired: 1 in, 2 out]
                              }
                              frame True {
                                n180 = property on="Tau 2" class="WFChart (strict)"("Active Plot"=u32 4) -> (error out=w540:errorcluster)  [unwired: 2 in, 1 out]
                                n181 = property on="Tau 2" class="WFChart (strict)"(error in=w540, "Plot.Visible?"=w538) -> ()  [unwired: 1 in, 2 out]
                                n182 = property on="g2" class="XYGraph (strict)"("Active Plot"=u32 4) -> (error out=w541:errorcluster)  [unwired: 2 in, 1 out]
                                n183 = property on="g2" class="XYGraph (strict)"(error in=w541, "Plot.Visible?"=w538) -> ()  [unwired: 1 in, 2 out]
                              }
                            }
                            n184 = case shown="False" w444 {
                              selector: w444 -> [w573 w578]
                              frame False {
                                n185 = property on="Tau 2" class="WFChart (strict)"("Active Plot"=u32 0) -> (error out=w574:errorcluster)  [unwired: 2 in, 1 out]
                                n186 = property on="g2" class="XYGraph (strict)"("Active Plot"=u32 0) -> (error out=w576:errorcluster)  [unwired: 2 in, 1 out]
                                n187 = property on="g2" class="XYGraph (strict)"(error in=w576, "Plot.Visible?"=w573) -> ()  [unwired: 1 in, 2 out]
                                n188 = property on="Tau 2" class="WFChart (strict)"(error in=w574, "Plot.Visible?"=w573) -> ()  [unwired: 1 in, 2 out]
                              }
                              frame True {
                                n189 = property on="Tau 2" class="WFChart (strict)"("Active Plot"=u32 0) -> (error out=w580:errorcluster)  [unwired: 2 in, 1 out]
                                n190 = property on="Tau 2" class="WFChart (strict)"(error in=w580, "Plot.Visible?"=w578) -> ()  [unwired: 1 in, 2 out]
                                n191 = property on="g2" class="XYGraph (strict)"("Active Plot"=u32 0) -> (error out=w581:errorcluster)  [unwired: 2 in, 1 out]
                                n192 = property on="g2" class="XYGraph (strict)"(error in=w581, "Plot.Visible?"=w578) -> ()  [unwired: 1 in, 2 out]
                              }
                            }
                            n193 = case shown="False" w439 {
                              selector: w439 -> [w523 w528]
                              frame False {
                                n194 = property on="Tau 2" class="WFChart (strict)"("Active Plot"=u32 5) -> (error out=w525:errorcluster)  [unwired: 2 in, 1 out]
                                n195 = property on="g2" class="XYGraph (strict)"("Active Plot"=u32 5) -> (error out=w526:errorcluster)  [unwired: 2 in, 1 out]
                                n196 = property on="g2" class="XYGraph (strict)"(error in=w526, "Plot.Visible?"=w523) -> ()  [unwired: 1 in, 2 out]
                                n197 = property on="Tau 2" class="WFChart (strict)"(error in=w525, "Plot.Visible?"=w523) -> ()  [unwired: 1 in, 2 out]
                              }
                              frame True {
                                n198 = property on="Tau 2" class="WFChart (strict)"("Active Plot"=u32 5) -> (error out=w529:errorcluster)  [unwired: 2 in, 1 out]
                                n199 = property on="Tau 2" class="WFChart (strict)"(error in=w529, "Plot.Visible?"=w528) -> ()  [unwired: 1 in, 2 out]
                                n200 = property on="g2" class="XYGraph (strict)"("Active Plot"=u32 5) -> (error out=w531:errorcluster)  [unwired: 2 in, 1 out]
                                n201 = property on="g2" class="XYGraph (strict)"(error in=w531, "Plot.Visible?"=w528) -> ()  [unwired: 1 in, 2 out]
                              }
                            }
                            n202 = case shown="False" w429 {
                              selector: w429 -> [w563 w568]
                              frame False {
                                n203 = property on="Tau 2" class="WFChart (strict)"("Active Plot"=u32 1) -> (error out=w565:errorcluster)  [unwired: 2 in, 1 out]
                                n204 = property on="g2" class="XYGraph (strict)"("Active Plot"=u32 1) -> (error out=w566:errorcluster)  [unwired: 2 in, 1 out]
                                n205 = property on="g2" class="XYGraph (strict)"(error in=w566, "Plot.Visible?"=w563) -> ()  [unwired: 1 in, 2 out]
                                n206 = property on="Tau 2" class="WFChart (strict)"(error in=w565, "Plot.Visible?"=w563) -> ()  [unwired: 1 in, 2 out]
                              }
                              frame True {
                                n207 = property on="Tau 2" class="WFChart (strict)"("Active Plot"=u32 1) -> (error out=w570:errorcluster)  [unwired: 2 in, 1 out]
                                n208 = property on="Tau 2" class="WFChart (strict)"(error in=w570, "Plot.Visible?"=w568) -> ()  [unwired: 1 in, 2 out]
                                n209 = property on="g2" class="XYGraph (strict)"("Active Plot"=u32 1) -> (error out=w571:errorcluster)  [unwired: 2 in, 1 out]
                                n210 = property on="g2" class="XYGraph (strict)"(error in=w571, "Plot.Visible?"=w568) -> ()  [unwired: 1 in, 2 out]
                              }
                            }
                            n211 = case shown="False" w438 {
                              selector: w438 -> [w513 w518]
                              frame False {
                                n212 = property on="Tau 2" class="WFChart (strict)"("Active Plot"=u32 6) -> (error out=w515:errorcluster)  [unwired: 2 in, 1 out]
                                n213 = property on="g2" class="XYGraph (strict)"("Active Plot"=u32 6) -> (error out=w516:errorcluster)  [unwired: 2 in, 1 out]
                                n214 = property on="g2" class="XYGraph (strict)"(error in=w516, "Plot.Visible?"=w513) -> ()  [unwired: 1 in, 2 out]
                                n215 = property on="Tau 2" class="WFChart (strict)"(error in=w515, "Plot.Visible?"=w513) -> ()  [unwired: 1 in, 2 out]
                              }
                              frame True {
                                n216 = property on="Tau 2" class="WFChart (strict)"("Active Plot"=u32 6) -> (error out=w519:errorcluster)  [unwired: 2 in, 1 out]
                                n217 = property on="Tau 2" class="WFChart (strict)"(error in=w519, "Plot.Visible?"=w518) -> ()  [unwired: 1 in, 2 out]
                                n218 = property on="g2" class="XYGraph (strict)"("Active Plot"=u32 6) -> (error out=w521:errorcluster)  [unwired: 2 in, 1 out]
                                n219 = property on="g2" class="XYGraph (strict)"(error in=w521, "Plot.Visible?"=w518) -> ()  [unwired: 1 in, 2 out]
                              }
                            }
                            n220 = case shown="False" w442 {
                              selector: w442 -> [w553 w558]
                              frame False {
                                n221 = property on="Tau 2" class="WFChart (strict)"("Active Plot"=u32 2) -> (error out=w554:errorcluster)  [unwired: 2 in, 1 out]
                                n222 = property on="g2" class="XYGraph (strict)"("Active Plot"=u32 2) -> (error out=w556:errorcluster)  [unwired: 2 in, 1 out]
                                n223 = property on="g2" class="XYGraph (strict)"(error in=w556, "Plot.Visible?"=w553) -> ()  [unwired: 1 in, 2 out]
                                n224 = property on="Tau 2" class="WFChart (strict)"(error in=w554, "Plot.Visible?"=w553) -> ()  [unwired: 1 in, 2 out]
                              }
                              frame True {
                                n225 = property on="Tau 2" class="WFChart (strict)"("Active Plot"=u32 2) -> (error out=w560:errorcluster)  [unwired: 2 in, 1 out]
                                n226 = property on="Tau 2" class="WFChart (strict)"(error in=w560, "Plot.Visible?"=w558) -> ()  [unwired: 1 in, 2 out]
                                n227 = property on="g2" class="XYGraph (strict)"("Active Plot"=u32 2) -> (error out=w561:errorcluster)  [unwired: 2 in, 1 out]
                                n228 = property on="g2" class="XYGraph (strict)"(error in=w561, "Plot.Visible?"=w558) -> ()  [unwired: 1 in, 2 out]
                              }
                            }
                            n229 = Wait (ms)(milliseconds to wait="Update Time (ms)\nDO NOT CHANGE!") -> ()  [unwired: 1 out]
                            n230 = call "UpdateData.vi"("Duration Time (ms)"="Integration Time (ms)", "Detector Select"=w428, "Delay Time"=w455) -> ("Elapsed Time(s)"=w456:sgl, "Intensity Array"=w454:sgl[], "Tau Array"=w453:sgl[], "mean"=w418:dbl, "mean 8"=w398:dbl, "mean 2"=w367:dbl, "mean 7"=w399:dbl, "mean 3"=w403:dbl, "Intensity data"=w452:string, "g2 Display"=→"g2":cluster{"Delay Time":sgl[], sgl[]}[], "mean 4"=w402:dbl, "mean 5"=w401:dbl, "mean 6"=w400:dbl, "tau data"=w422:string, "g2 data"=w423:string)  [unwired: 2 in]
                            n231 = Multiply(x=sgl 1000.0, y=w456) -> (x*y=w460:sgl)
                            n232 = Less?(x=w418, y=1.005) -> (x < y?=w397:bool)
                            n233 = Less?(x=w367, y=1.005) -> (x < y?=w351:bool)
                            n234 = Less?(x=w403, y=1.005) -> (x < y?=w350:bool)
                            n235 = Less?(x=w402, y=1.005) -> (x < y?=w347:bool)
                            n236 = Less?(x=w401, y=1.005) -> (x < y?=w345:bool)
                            n237 = Less?(x=w400, y=1.005) -> (x < y?=w343:bool)
                            n238 = Less?(x=w399, y=1.005) -> (x < y?=w341:bool)
                            n239 = Less?(x=w398, y=1.005) -> (x < y?=w339:bool)
                            n240 = Index Array(array=w454, index #1=0, index #2=1, index #3=2, index #4=3, index #5=4, index #6=5, index #7=6, index #8=7) -> (element #1=w395:sgl, element #2=w374:sgl, element #3=w373:sgl, element #4=w372:sgl, element #5=w371:sgl, element #6=w370:sgl, element #7=w369:sgl, element #8=w368:sgl)
                            "Det 7" <- w369
                            "Det 6" <- w370
                            "Det 5" <- w371
                            "Det 4" <- w372
                            "Det 3" <- w373
                            "Det 2" <- w374
                            "Det 1" <- w395
                            "Det 8" <- w368
                            n241 = Subtract(x="Integration Time (ms)", y=w460) -> (x-y=w458:sgl)
                            "Time Left (ms)" <- w458
                            n242 = Greater?(x=w418, y=0.98) -> (0:w396:bool)
                            n243 = Greater?(x=w402, y=0.98) -> (0:w348:bool)
                            n244 = Greater?(x=w400, y=0.98) -> (0:w344:bool)
                            n245 = Greater?(x=w398, y=0.98) -> (0:w340:bool)
                            n246 = Greater Or Equal?(x=w395, y=sgl 2.0) -> (x >= y?=w392:bool)
                            n247 = Greater Or Equal?(x=w374, y=sgl 2.0) -> (x >= y?=w338:bool)
                            n248 = Greater Or Equal?(x=w373, y=sgl 2.0) -> (x >= y?=w336:bool)
                            n249 = Greater Or Equal?(x=w372, y=sgl 2.0) -> (x >= y?=w334:bool)
                            n250 = Greater Or Equal?(x=w371, y=sgl 2.0) -> (x >= y?=w332:bool)
                            n251 = Greater Or Equal?(x=w370, y=sgl 2.0) -> (x >= y?=w330:bool)
                            n252 = Less Or Equal?(x=w395, y=sgl 1000.0) -> (x <= y?=w391:bool)
                            n253 = Less Or Equal?(x=w374, y=sgl 1000.0) -> (x <= y?=w337:bool)
                            n254 = Less Or Equal?(x=w373, y=sgl 1000.0) -> (x <= y?=w335:bool)
                            n255 = Less Or Equal?(x=w372, y=sgl 1000.0) -> (x <= y?=w333:bool)
                            n256 = Less Or Equal?(x=w371, y=sgl 1000.0) -> (x <= y?=w331:bool)
                            n257 = Less Or Equal?(x=w370, y=sgl 1000.0) -> (x <= y?=w329:bool)
                            n258 = Less Or Equal?(x=w369, y=sgl 1000.0) -> (x <= y?=w327:bool)
                            n259 = Less Or Equal?(x=w368, y=sgl 1000.0) -> (x <= y?=w325:bool)
                            n260 = Greater Or Equal?(x=w369, y=sgl 2.0) -> (x >= y?=w328:bool)
                            n261 = Greater Or Equal?(x=w368, y=sgl 2.0) -> (x >= y?=w326:bool)
                            n262 = Greater?(x=w367, y=0.98) -> (0:w352:bool)
                            n263 = Greater?(x=w403, y=0.98) -> (0:w349:bool)
                            n264 = Greater?(x=w401, y=0.98) -> (0:w346:bool)
                            n265 = Greater?(x=w399, y=0.98) -> (0:w342:bool)
                            n266 = Build Array(w397, w396, w392, w391) -> (w390:bool[])
                            n267 = Build Array(w352, w351, w338, w337) -> (w366:bool[])
                            n268 = Build Array(w350, w349, w336, w335) -> (w365:bool[])
                            n269 = Build Array(w348, w347, w334, w333) -> (w364:bool[])
                            n270 = Build Array(w346, w345, w332, w331) -> (w363:bool[])
                            n271 = Build Array(w344, w343, w330, w329) -> (w362:bool[])
                            n272 = Build Array(w342, w341, w328, w327) -> (w361:bool[])
                            n273 = Build Array(w340, w339, w326, w325) -> (w360:bool[])
                            n274 = And Array Elements(Boolean array=w390) -> (logical AND=w389:bool)
                            n275 = And Array Elements(Boolean array=w366) -> (logical AND=w353:bool)
                            n276 = And Array Elements(Boolean array=w365) -> (logical AND=w354:bool)
                            n277 = And Array Elements(Boolean array=w364) -> (logical AND=w355:bool)
                            n278 = And Array Elements(Boolean array=w363) -> (logical AND=w356:bool)
                            n279 = And Array Elements(Boolean array=w362) -> (logical AND=w357:bool)
                            n280 = And Array Elements(Boolean array=w361) -> (logical AND=w358:bool)
                            n281 = And Array Elements(Boolean array=w360) -> (logical AND=w359:bool)
                            n282 = Less Or Equal To 0?(x=w458) -> (x <= 0?=w459:bool)
                            n283 = case shown="True" w389 {
                              frame False {
                                n284 = control-ref of="Det 1"() -> (w492:refnum<vi>)
                                n285 = property on="Property Node" class="Digital (strict)"(reference=w492, "DisabledEnum"=T4."Disabled and Grayed Out" ("Disabled")) -> ()  [unwired: 1 in, 2 out]
                              }
                              frame True {
                                n286 = control-ref of="Det 1"() -> (w494:refnum<vi>)
                                n287 = property on="Property Node" class="Digital (strict)"(reference=w494, "DisabledEnum"=T4."Enabled" ("Disabled")) -> ()  [unwired: 1 in, 2 out]
                              }
                            }
                            n288 = case shown="True" w353 {
                              frame False {
                                n289 = control-ref of="Det 2"() -> (w488:refnum<vi>)
                                n290 = property on="Property Node" class="Digital (strict)"(reference=w488, "DisabledEnum"=T4."Disabled and Grayed Out" ("Disabled")) -> ()  [unwired: 1 in, 2 out]
                              }
                              frame True {
                                n291 = control-ref of="Det 2"() -> (w490:refnum<vi>)
                                n292 = property on="Property Node" class="Digital (strict)"(reference=w490, "DisabledEnum"=T4."Enabled" ("Disabled")) -> ()  [unwired: 1 in, 2 out]
                              }
                            }
                            n293 = case shown="True" w354 {
                              frame False {
                                n294 = control-ref of="Det 3"() -> (w484:refnum<vi>)
                                n295 = property on="Property Node" class="Digital (strict)"(reference=w484, "DisabledEnum"=T4."Disabled and Grayed Out" ("Disabled")) -> ()  [unwired: 1 in, 2 out]
                              }
                              frame True {
                                n296 = control-ref of="Det 3"() -> (w486:refnum<vi>)
                                n297 = property on="Property Node" class="Digital (strict)"(reference=w486, "DisabledEnum"=T4."Enabled" ("Disabled")) -> ()  [unwired: 1 in, 2 out]
                              }
                            }
                            n298 = case shown="True" w355 {
                              frame False {
                                n299 = control-ref of="Det 4"() -> (w480:refnum<vi>)
                                n300 = property on="Property Node" class="Digital (strict)"(reference=w480, "DisabledEnum"=T4."Disabled and Grayed Out" ("Disabled")) -> ()  [unwired: 1 in, 2 out]
                              }
                              frame True {
                                n301 = control-ref of="Det 4"() -> (w482:refnum<vi>)
                                n302 = property on="Property Node" class="Digital (strict)"(reference=w482, "DisabledEnum"=T4."Enabled" ("Disabled")) -> ()  [unwired: 1 in, 2 out]
                              }
                            }
                            n303 = case shown="True" w356 {
                              frame False {
                                n304 = control-ref of="Det 5"() -> (w476:refnum<vi>)
                                n305 = property on="Property Node" class="Digital (strict)"(reference=w476, "DisabledEnum"=T4."Disabled and Grayed Out" ("Disabled")) -> ()  [unwired: 1 in, 2 out]
                              }
                              frame True {
                                n306 = control-ref of="Det 5"() -> (w478:refnum<vi>)
                                n307 = property on="Property Node" class="Digital (strict)"(reference=w478, "DisabledEnum"=T4."Enabled" ("Disabled")) -> ()  [unwired: 1 in, 2 out]
                              }
                            }
                            n308 = case shown="False" w357 {
                              frame False {
                                n309 = control-ref of="Det 6"() -> (w472:refnum<vi>)
                                n310 = property on="Property Node" class="Digital (strict)"(reference=w472, "DisabledEnum"=T4."Disabled and Grayed Out" ("Disabled")) -> ()  [unwired: 1 in, 2 out]
                              }
                              frame True {
                                n311 = control-ref of="Det 6"() -> (w474:refnum<vi>)
                                n312 = property on="Property Node" class="Digital (strict)"(reference=w474, "DisabledEnum"=T4."Enabled" ("Disabled")) -> ()  [unwired: 1 in, 2 out]
                              }
                            }
                            n313 = case shown="True" w358 {
                              frame False {
                                n314 = control-ref of="Det 7"() -> (w468:refnum<vi>)
                                n315 = property on="Property Node" class="Digital (strict)"(reference=w468, "DisabledEnum"=T4."Disabled and Grayed Out" ("Disabled")) -> ()  [unwired: 1 in, 2 out]
                              }
                              frame True {
                                n316 = control-ref of="Det 7"() -> (w470:refnum<vi>)
                                n317 = property on="Property Node" class="Digital (strict)"(reference=w470, "DisabledEnum"=T4."Enabled" ("Disabled")) -> ()  [unwired: 1 in, 2 out]
                              }
                            }
                            n318 = case shown="True" w359 {
                              frame False {
                                n319 = control-ref of="Det 8"() -> (w464:refnum<vi>)
                                n320 = property on="Property Node" class="Digital (strict)"(reference=w464, "DisabledEnum"=T4."Disabled and Grayed Out" ("Disabled")) -> ()  [unwired: 1 in, 2 out]
                              }
                              frame True {
                                n321 = control-ref of="Det 8"() -> (w466:refnum<vi>)
                                n322 = property on="Property Node" class="Digital (strict)"(reference=w466, "DisabledEnum"=T4."Enabled" ("Disabled")) -> ()  [unwired: 1 in, 2 out]
                              }
                            }
                            n323 = Or(x=w426, y=w459) -> (x .or. y?=w457:bool)
                            n324 = case shown="True" w457 {
                              tunnel: w428 -> [w583 _]
                              frame True {
                                n325 = case shown="\"8 Detectors\", Default" w583 {
                                frame "4 Detectors" {
                                n326 = dll-call lib="C:/Users/BUCKLEY-ADMIN/Desktop/DCScode_simulISS_MAP/flex05-4chPascal.dll" fn="USBStop" label="StopCH4"() -> ()  [unwired: 4 in, 2 out]
                                }
                                frame "8 Detectors", Default {
                                n327 = dll-call lib="C:/Users/BUCKLEY-ADMIN/Desktop/DCScode_simulISS_MAP/flex05oem8chauto100nsPASCAL_win7.dll" fn="USBStop" label="StopCH8"() -> ()  [unwired: 4 in, 2 out]
                                }
                                }
                              }
                              frame False {
                              }
                            }
                          }
                          n328 = local read "Trial #"() -> (w261:u32)
                          n329 = property on="QUIT" class="Bool"("Disabled"=w242) -> ()  [unwired: 2 in, 2 out]
                          n330 = Increment(x=w261) -> (x+1=w260:u32)
                          n331 = property on="Sequence Scan" class="Bool"("Disabled"=w242) -> ()  [unwired: 2 in, 2 out]
                          n332 = local write "Trial #"(w260) -> ()
                          n333 = property on="Update Time (ms)\nDO NOT CHANGE!" class="DigNum (strict)"("Disabled"=w242) -> ()  [unwired: 2 in, 2 out]
                          n334 = property on="Integration Time (ms)" class="DigNum (strict)"("Disabled"=w242) -> ()  [unwired: 2 in, 2 out]
                          n335 = property on="Detector Select" class="RadioBtnsControl (strict)"("Disabled"=w242) -> ()  [unwired: 2 in, 2 out]
                          n336 = property on="Initialize Correlator" class="Bool"("Disabled"=w242) -> ()  [unwired: 2 in, 2 out]
                          n337 = case shown="\"Det 2\"" "Detector Used" {
                            tunnel: [1 2 3 4 5 6 7 8] -> w263
                            frame "Det 1", Default {
                            }
                            frame "Det 2" {
                            }
                            frame "Det 3" {
                            }
                            frame "Det 4" {
                            }
                            frame "Det 5" {
                            }
                            frame "Det 6" {
                            }
                            frame "Det 7" {
                            }
                            frame "Det 8" {
                            }
                          }
                          n338 = for {
                            N: 1 -> [_]
                            tunnel: w269 -> [w313]
                            tunnel: [w316] -> w249
                            tunnel: w263 -> [w315]
                            tunnel: w258 -> [w306]
                            n339 = Index Array(array=w313, index=w315) -> (element=w314:sgl)
                            n340 = Boolean To (0,1)(Boolean="Baseline") -> (0, 1=w318:i16)
                            n341 = case shown="True" w306 {
                              tunnel: [0.0 w320] -> w310
                              tunnel: inf -> [_ w320]
                              frame False {
                              }
                              frame True {
                              }
                            }
                            n342 = case shown="True" w306 {
                              tunnel: [u32 0 w322] -> w316
                              frame False {
                              }
                              frame True {
                                n343 = local read "Mark #"() -> (w324:u32)
                                n344 = local write "Trial #"(u32 0) -> ()
                                n345 = Increment(x=w324) -> (x+1=w322:u32)
                                n346 = local write "Mark #"(w322) -> ()
                              }
                            }
                            n347 = feedback #1() -> (w311:sgl)  [unwired: 1 in]
                            n348 = formula code="if(Tau==0) Tau=Tau+0.001;\nif(T==1) baselineflow=Tau;\n\ntmp=baselineflow/Tau;"("Tau"=w314, "T"=w318, "baselineflow"=w311) -> ("tmp"=w308:dbl, "baselineflow"=w312:sgl)
                            n349 = feedback-in #1(w312) -> ()
                            n350 = Bundle("tmp"=w308, w310) -> (→"Tau":cluster{"tmp":dbl, dbl})  [unwired: 1 in]
                          }
                          n351 = property on="Frame #" class="DigNum (strict)"() -> ("Value"=w252:u32)  [unwired: 2 in, 2 out]
                          n352 = case shown="True" "Fixed Time" {
                            tunnel: w252 -> [w294 w297]
                            tunnel: [w294 w297] -> w243
                            frame False {
                            }
                            frame True {
                              n353 = Less Or Equal?(x="Fixed # of Frames", y=w297) -> (x <= y?=w295:bool)
                              n354 = local write "Stop"(w295) -> ()
                            }
                          }
                          n355 = case shown="\"8 Detectors\", Default" w241 {
                            tunnel: w249 -> [w591 w595]
                            tunnel: [w592 w594] -> w278
                            tunnel: [4 8] -> w257
                            frame "4 Detectors" {
                              n356 = Build Array(w591, w591, w591, w591, w591) -> (w592:u32[])
                            }
                            frame "8 Detectors", Default {
                              n357 = Build Array(w595, w595, w595, w595, w595, w595, w595, w595, w595) -> (w594:u32[])
                            }
                          }
                          n358 = Increment(x=w243) -> (x+1=w253:u32)
                          n359 = local write "Frame #"(w253) -> ()
                          n360 = case shown="\"8 Detectors\", Default" w241 {
                            tunnel: ["%Duration\tID1\t\tID2\t\tID3\t\tID4\n" "%Duration\tID1\t\tID2\t\tID3\t\tID4\t\tID5\t\tID6\t\tID7\t\tID8\n"] -> w275
                            tunnel: ["%Tau\t\tTau1\t\tTau2\t\tTau3\t\tTau4\n" "%Tau\t\tTau1\t\tTau2\t\tTau3\t\tTau4\t\tTau5\t\tTau6\t\tTau7\t\tTau8\n"] -> w274
                            tunnel: ["%Delaytime\tD1\t\tD2\t\tD3\t\tD4\n" "%Delaytime\tD1\t\tD2\t\tD3\t\tD4\t\tD5\t\tD6\t\tD7\t\tD8\n"] -> w273
                            frame "4 Detectors" {
                            }
                            frame "8 Detectors", Default {
                            }
                          }
                          n361 = Number To Decimal String(number=w243) -> (decimal integer string=w279:string)  [unwired: 1 in]
                          n362 = Get Date/Time In Seconds() -> (seconds since 1Jan1904=w287:timestamp)
                          n363 = Array To Spreadsheet String(array=w278, 3:"%d") -> (spreadsheet string=w276:string)  [unwired: 1 in]
                          n364 = Format Date/Time String(seconds (now)=w287) -> (date/time string=w284:string)  [unwired: 2 in]
                          "Computer Time" <- w284
                          n365 = Concatenate Strings("File Name:", "_flow_", w279, ".dat") -> (w255:string)
                          n366 = Build Path(base path="Data Save Directory:", name or relative path=w255) -> (appended path=w247:path)
                          n367 = local read "Test"() -> (w251:bool)
                          n368 = Concatenate Strings("%", w284, "\r\n", w275, w272, w274, "%\t\t", w271, w273, w270, w276) -> (w259:string)
                          n369 = case shown="False" w251 {
                            tunnel: w259 -> [w291 _]
                            tunnel: w247 -> [w290 _]
                            tunnel: [w289 _] -> w246
                            tunnel: [w288 _] -> w245
                            frame False {
                              n370 = Write to Text File(file (use dialog)=w290, text=w291) -> (refnum out=w292:refnum<file>, error out=w293:errorcluster)  [unwired: 2 in, 1 out]
                              n371 = Close File(refnum=w292, error in=w293) -> (path=w289:path, error out=w288:errorcluster)
                            }
                            frame True {
                            }
                          }
                        }
                      }
                      n372 = local read "Test"() -> (w171:bool)
                      n373 = for {
                        N: 1 -> [_]
                        tunnel: w198 -> [_]
                        n374 = local write "Stop"(FALSE) -> ()
                        n375 = Wait (ms)(milliseconds to wait="Delay between frames(ms)") -> ()  [unwired: 1 out]
                      }
                      n376 = Unbundle By Name(w178) -> ("status"=w197:bool)
                      n377 = Not(x=w171) -> (.not. x?=w166:bool)
                      n378 = Not(x=w197) -> (.not. x?=w196:bool)
                      n379 = And(x="Real Time Fitting?", y=w166) -> (x .and. y?=w170:bool)
                      n380 = case shown="True" w170 {
                        tunnel: w196 -> [_ w205]
                        tunnel: w177 -> [_ w204]
                        tunnel: w176 -> [_ w203]
                        tunnel: w173 -> [w200 w202]
                        tunnel: [w200 w201] -> w172
                        frame False {
                        }
                        frame True {
                          n381 = case shown="True" w205 {
                            tunnel: w204 -> [_ w225]
                            tunnel: w203 -> [_ w221]
                            tunnel: w202 -> [w206 w217]
                            tunnel: [w206 w215] -> w201
                            frame False {
                            }
                            frame True {
                              # "Initialize Array of NaNs with size of \"fixed number of frames, \nand run this array into the case structure by putting it \nthrough a shift register with each loop it will replace one of \nthe NaNs by the flow data of the detector used. Then this data\nis averaged and COV is calculated."
                              n382 = property on="Data Save Directory:" class="Path"() -> ("Value"=w227:path)  [unwired: 2 in, 2 out]
                              n383 = property on="File Name:" class="Str"() -> ("Value"=w228:string)  [unwired: 2 in, 2 out]
                              n384 = call "GetFilePath.vi"("path"=w227, "file name"=w228, "frame number"=w225) -> ("final path C"=w220:string)  [unwired: 10 in, 2 out]
                              n385 = property on="Avg" class="Arr (strict)"() -> ("Value"=w226:bool[][])  [unwired: 2 in, 2 out]
                              n386 = call "DCSAnalysis.vi"("# Detectors"=w221, "File path"=w220, "Frame #"=w225, "rho"="rho", "other settings"="Other Settings", "avgBool"=w226, "var values"="Initial Guess") -> ("Flow in each detector"=w218:dbl[], "Tau"=→"Tau 2":T3)  [unwired: 18 in, 1 out]
                              "Flow in each detector" <- w218
                              n387 = local read "Detector Used"() -> (w208:T2)
                              n388 = local read "Trial #"() -> (w213:u32)
                              n389 = Decrement(x=w213) -> (x-1=w214:u32)
                              n390 = Index Array(array=w218, index=w208) -> (element=w216:dbl)
                              n391 = Replace Array Subset(array=w217, new element=w216, index=w214) -> (w215:dbl[])
                              n392 = call <vilib>:"Std Deviation and Variance.vi"("X"=w215) -> ("mean"=w211:dbl, "standard deviation"=w212:dbl)  [unwired: 1 in, 1 out]
                              "mean" <- w211
                              n393 = Divide(x=w212, y=w211) -> (x/y=w210:dbl)
                              n394 = Multiply(x=w210, y=100.0) -> (x*y=→"COV":dbl)
                            }
                          }
                        }
                      }
                    }
                    n395 = call "iBs.vi"("Laser On/Off"=TRUE, "VISA resource name"="Laser Input Name") -> ()
                    n396 = Build Array(FALSE) -> (w152:bool[])
                    n397 = call "DAQ Assistant7"("data"=w152) -> ()  [unwired: 17 in, 2 out]
                    n398 = local read "Test"() -> (w146:bool)
                    n399 = case shown="False" w146 {
                      frame False {
                        # "This bit stores the time stamp."
                        n400 = local read "File Name:"() -> (w156:string)
                        n401 = Get Date/Time In Seconds() -> (seconds since 1Jan1904=w158:timestamp)
                        n402 = local read "Data Save Directory:"() -> (w157:path)
                        n403 = Format Date/Time String(seconds (now)=w158) -> (date/time string=w164:string)  [unwired: 2 in]
                        n404 = Concatenate Strings(w156, "_TIMING", ".dat") -> (w161:string)
                        n405 = Build Path(base path=w157, name or relative path=w161) -> (appended path=w160:path)
                        n406 = Write to Text File(file (use dialog)=w160, text=w164) -> (refnum out=w163:refnum<file>, error out=w162:errorcluster)  [unwired: 2 in, 1 out]
                        n407 = Close File(refnum=w163, error in=w162) -> ()  [unwired: 2 out]
                      }
                      frame True {
                      }
                    }
                  }
                  frame True {
                    n408 = invoke on="Sequence Scan" class="Bool" method="Reinit To Default"() -> ()  [unwired: 3 in, 3 out]
                    n409 = call "Display Message to User5"() -> ()  [unwired: 10 in, 2 out]
                  }
                }
              }
            }
            "Frame #" <- u32 0
            "Mark #" <- u32 0
            "Trial #" <- u32 0
          }
          event "QUIT": Value Change {
            # "Reset correlator before quitting"
            n410 = event-data() -> ()  [unwired: 1 in, 6 out]
            n411 = local write "Status"("Quit") -> ()
            n412 = case shown="\"8 Detectors\", Default" w604 {
              frame "4 Detectors" {
                n413 = dll-call lib="C:/Users/BUCKLEY-ADMIN/Desktop/DCScode_simulISS_MAP/flex05-4chPascal.dll" fn="USBInitialize" label="InitCH4"() -> (error out=w605:errorcluster)  [unwired: 4 in, 1 out]
                n414 = dll-call lib="C:/Users/BUCKLEY-ADMIN/Desktop/DCScode_simulISS_MAP/flex05-4chPascal.dll" fn="USBFree" label="FreeCH4"(error in=w605) -> ()  [unwired: 3 in, 2 out]
              }
              frame "8 Detectors", Default {
                n415 = dll-call lib="C:/Users/BUCKLEY-ADMIN/Desktop/DCScode_simulISS_MAP/flex05oem8chauto100nsPASCAL_win7.dll" fn="USBInitialize" label="InitCH8"() -> (error out=w606:errorcluster)  [unwired: 4 in, 1 out]
                n416 = dll-call lib="C:/Users/BUCKLEY-ADMIN/Desktop/DCScode_simulISS_MAP/flex05oem8chauto100nsPASCAL_win7.dll" fn="USBFree" label="FreeCH8"(error in=w606) -> ()  [unwired: 3 in, 2 out]
              }
            }
            n417 = local write "Status"("Quit") -> ()
          }
          event Timeout {
            w611 = TRUE
            w610 = u8 0
            # "This case structure turns on\n      and off the ISS Lasers"
            # "This case structure ensures that when the\noptical switch is turned on, the relay tells \nthe laser to power on."
            # "The system sits here and wait for some buttons to be pressed. And the status is always \"waiting\". Once some button is pressed, this value driven event\nstructure goes to the appropriate frame."
            n418 = event-data() -> ()  [unwired: 1 in, 3 out]
            n419 = local write "Status"("Waiting") -> ()
            n420 = property on="MARK\nMark" class="Bool"("DisabledEnum"=w610) -> ()  [unwired: 2 in, 2 out]
            n421 = property on="QUIT" class="Bool"("Disabled"=w610) -> ()  [unwired: 2 in, 2 out]
            n422 = property on="Sequence Scan" class="Bool"("Disabled"=w610) -> ()  [unwired: 2 in, 2 out]
            n423 = property on="Initialize Correlator" class="Bool"("Disabled"=w610) -> ()  [unwired: 2 in, 2 out]
            n424 = property on="Update Time (ms)\nDO NOT CHANGE!" class="DigNum (strict)"("Disabled"=w610) -> ()  [unwired: 2 in, 2 out]
            n425 = property on="Integration Time (ms)" class="DigNum (strict)"("Disabled"=w610) -> ()  [unwired: 2 in, 2 out]
            n426 = property on="Detector Select" class="RadioBtnsControl (strict)"("Disabled"=w610) -> ()  [unwired: 2 in, 2 out]
            n427 = case shown="True" "ISS Lasers ON" {
              frame False {
                n428 = Build Array(FALSE) -> (w618:bool[])
                n429 = call "DAQ Assistant5"("data"=w618) -> ()  [unwired: 17 in, 2 out]
              }
              frame True {
                # "For Toptica laser control"
                n430 = local read "Laser Input Name"() -> (w620:refnum<visa-resource-name>)
                n431 = call "iBs.vi"("Laser On/Off"=TRUE, "VISA resource name"=w620) -> ()
                n432 = Build Array(TRUE) -> (w622:bool[])
                n433 = call "DAQ Assistant6"("data"=w622) -> ()  [unwired: 17 in, 2 out]
              }
            }
            n434 = case shown="True" "Optical Switch OPEN" {
              frame False {
                # "Send 2 signals, one for LED indicator, one for switch"
                n435 = Build Array(FALSE, FALSE) -> (w624:bool[])
                n436 = call "DAQ Assistant3"("data"=w624) -> ()  [unwired: 17 in, 2 out]
              }
              frame True {
                n437 = Build Array(TRUE, TRUE) -> (w627:bool[])
                n438 = call "DAQ Assistant4"("data"=w627) -> ()  [unwired: 17 in, 2 out]
              }
            }
            n439 = Current VI's Menubar() -> (w613:refnum<k9>)
            n440 = Set Menu Item Info(7:"File", 9:w611, 11:w613) -> (3:w612:refnum<k9>)  [unwired: 4 in, 1 out]
            n441 = Get Date/Time In Seconds() -> (seconds since 1Jan1904=w616:timestamp)
            n442 = Set Menu Item Info(7:"Options", 9:w611, 11:w612) -> ()  [unwired: 4 in, 2 out]
            n443 = Format Date/Time String(seconds (now)=w616) -> (date/time string=w617:string)  [unwired: 2 in]
            n444 = local write "Computer Time"(w617) -> ()
          }
        }
      }
    }
  }
  n445 = call "BioFeedbackEMG.vi"("stop"=w2, "Start"=TRUE) -> ("filtered signal (single sample)"=→"filtered signal (single sample)":waveform(dbl), "Data Levels"=→"Data Levels":dbl)  [unwired: 8 in]
